vi "HostMain.vi"() -> ()   [LabVIEW 2024]
uses:
  C:/Users/ROAR/Documents/Rob Motor Assessment stuff/Labview/RobUST_3D_with_Unity_Control_PXI_Low_Level_Only_Streamlined/Vicon_files/ViconDataStreamSDK_DotNET.dll
  Vicon_files/ViconDataStreamSDK_DotNET.dll
  typeDef/Modes_knees.ctl
  <vilib>/Platform/TimedLoop/XDataNode/timing_clust.ctl
  <vilib>/Platform/TimedLoop/XDataNode/nitl_modes.ctl
  <vilib>/Platform/TimedLoop/XDataNode/wakeup.ctl
  <vilib>/Utility/file.llb/Read Delimited Spreadsheet (DBL).vi
  <vilib>/platform/TimedLoop/XDataNode/XDataNode.xnode
  <vilib>/Utility/Variable/NI_VariableUtilities.lvlib
  <vilib>/Platform/TimedLoop/XDataNode/XDNodeRunTimeDep.lvlib
  <vilib>/Analysis/NI_AALBase.lvlib
panel:
  out "All tensions mean":dbl[](array[numeric])
  out "Captured tensions mean":dbl[](array[numeric])
  out "Captured tensions standard dev":dbl[](array[numeric])
  in  "Capture current tension mean and standard dev":bool
  out "All tensions standard dev":dbl[](array[numeric])
  out "All tensions history":dbl[][](array[numeric])
  in  "ConstantModeActiveMotorFlags":bool[](array[boolean])
  out "StartManualTensionRecordTimeInSeconds":dbl
  out "RecordTime (s)":dbl
  out "Manually record tensions flag previous state":bool
  in  "MaxTensionsRecordTimeInSecs":dbl
  in  "RecordTensionsForGivenTimeFlag":bool
  out "Task has ended flag":bool
  out "Tension tare values":dbl[](array[numeric])
  in  "Live plot tensions flag":bool
  out "New info string received":bool
  out "Unity task info string":string
  in  "Use sinusoid":bool
  in  "Sinusoid period (s)":dbl
  in  "Sinusoid amplitude (N)":dbl
  in  "Single motor number":i32
  in  "Single motor tension current set value":dbl=10.0 min=10.0
  in  "Single motor tension desired set value":dbl
  in  "Change constant tension value toggle":bool
  out "Finished Late? [i-1]":bool
  out "CablesTared?":bool
  out "Data to save":dbl[][](array[numeric])
  out "Current save file out":path
  out "Connected to Unity last save call?":bool
  in  "Constant mode cable tensions N":dbl
  out "Last Vicon Frame Read":u32
  out "LastTimeUnityTensionsReceivedInMs":u32
  out "TensionsUpdateRateHz":dbl
  out "UnityDesiredCableTensionsInAscendingOrder":dbl[](array[numeric])
  in  "Mode Robot":T1(radio)
  in  "Total Number Motors":i32
  out "Latest tensions":dbl[](array[numeric])
  in  "Tare":bool
  out "Trunk Structure Matrix":dbl[][](array[numeric])
  out "Trunk FF type specifier":string
  out "Center point for FF":dbl[](array[numeric])
  out "Excursion distances Vicon frame":dbl[](array[numeric])
  out "TCP connection to Unity?":bool
  out "Unity TCP connection ID":refnum<k5>
  out "Control point position coords":dbl[](array[numeric])
  in  "Control point data source":T2(radio)
  in  "perturbation directions":string
  in  "Refresh Center 2":bool
  in  "Insert Test Name":string
  out "CurrentPttrunk":cluster{dbl[], dbl[]}
  out "Centertrunk":cluster{dbl[], dbl[]}
  out "xyboundstrunk":cluster{dbl[], dbl[]}
  out "trunk markers":dbl[](array[numeric])
  out "pel markers":dbl[](array[numeric])
  out "whichMode 3":bool[](array[boolean])
  in  "Mode Knees":T3
  out "whichMode 2":bool[](array[boolean])
  in  "?":enum32{"Trunk FF", "Pelvis FF"}(tab)
  in  "Turn On":bool
  out "Trunk Graph":cluster{dbl[], dbl[]}[](graph)
  out "Pelvis Graph":cluster{dbl[], dbl[]}[](graph)
  in  "Turn On Pelv":bool
  out "PelvisGraphyz":cluster{dbl[], dbl[]}[](graph)
  in  "?":T4(tab)
  in  "% Body Weight":dbl=10.0
  in  "FM --- FF":dbl[](array[numeric])=[30.0, 15.0, 15.0, 15.0, 2.0, 2.0]
  in  "Force Field Radius (m)":dbl=0.05
  in  "Update R or FF":bool
  in  "Refresh Center":bool
  in  "Select File with Trunk\nBoundary Points":path=path "" caption="start path"
  in  "Pert Reset":bool
  in  "Apply Pert":bool
  out "Weight [lbs]":dbl
  in  "Update Pert Parameters":bool
  in  "Pert Direction":i16(knob) scale=0.0..7.0
  in  "Rise Time":dbl
  in  "Constant Time":dbl
  in  "Fall Time":dbl
  in  "Amp [%BW]":dbl
  in  "Weight [Kg]":dbl
  in  "Mode Pelvis":enum32{"Idle", "Constant", "Force", "Pert"}(radio)
  out "Boolean":bool
  out "14":cluster{"[0]":dbl, "[1]":dbl}(graph)
  out "13":cluster{"[0]":dbl, "[1]":dbl}(graph)
  out "12":cluster{"[0]":dbl, "[1]":dbl}(graph)
  out "11":cluster{"[0]":dbl, "[1]":dbl}(graph)
  out "10":cluster{"[0]":dbl, "[1]":dbl}(graph)
  out "9":cluster{"[0]":dbl, "[1]":dbl}(graph)
  in  "?":T5(tab)
  in  "Reset Label":bool
  out "Going Up":bool
  in  "record trajectory":bool
  in  "Weight (Kg) --- FF 2":dbl=50.0
  in  "% Body Weight 2":dbl=10.0
  in  "FM --- FF 2":dbl[](array[numeric])=[30.0, 5.0, 5.0, 5.0, 2.0, 2.0]
  in  "Update R or FF 2":bool
  in  "Pelvis Radius FF":dbl=0.03
  in  "Weight [Kg] 3":dbl=75.0
  in  "Amp [%BW] 3":dbl=10.0
  in  "Fall Time 2":dbl=200.0
  in  "Constant Time 2":dbl=200.0
  in  "Rise Time 2":dbl=200.0
  in  "Pert Direction 2":i16(knob) scale=0.0..7.0
  in  "Update Pert Parameters 2":bool
  out "Weight [lbs] 3":dbl
  in  "Apply Pert 2":bool
  in  "Pert Reset 2":bool
  in  "Set Unit Force Vector":dbl[](array[numeric])=[0.0, 0.0, -1.0, 15.0, 2.0, 2.0]
  in  "Update_setForces":bool
  in  "Set % Body Weight":dbl=10.0
  in  "Weight (lb)":dbl=50.0
  out "ATI":dbl[](graph)
  in  "ATI UnBias":bool
  in  "ATI Bias":bool
  out "Saving Data":bool
  out "whichMode":bool[](array[boolean])
  in  "pidGains":dbl[][](array[numeric])=[[3.5, 1.7, 3.0000000000000004, 1.7, 1.7, 3.5, 1.7, 1.7, 2.0, 1.7, 1.7, 3.0, 1.7, 3.5], [0.001, 0.003, 0.003, 0.001, 0.001, 0.003, 0.0008, 0.003, 0.001, 0.003, 0.001, 0.003, 0.001, 0.001], [0.0004, 0.0012, 0.0006, 0.0012, 0.0012, 0.0004, 0.0012, 0.0012, 0.0008, 0.0012, 0.0012, 0.0004, 0.0012, 0.0004]]
  in  "SetPID":bool
  out "4":cluster{"[0]":dbl, "[1]":dbl}(graph)
  out "3":cluster{"[0]":dbl, "[1]":dbl}(graph)
  out "2":cluster{"[0]":dbl, "[1]":dbl}(graph)
  out "1":cluster{"[0]":dbl, "[1]":dbl}(graph)
  out "8":cluster{"[0]":dbl, "[1]":dbl}(graph)
  out "7":cluster{"[0]":dbl, "[1]":dbl}(graph)
  out "6":cluster{"[0]":dbl, "[1]":dbl}(graph)
  out "FB n FF O/P(N)":dbl[](graph)
  out "Current Filename":string
  out ".NET Reference out":refnum<k24>
  out "ViconTab":enum32{"Vicon", "no Vicon"}(tab)
  out "Frame Number":dbl format="%.2f"
  out "Subject Name":string
  out "Markers Count":u32
  in  "Connect\nVicon":bool
  in  "Update\nMarkers":bool
  in  "Vicon Static":bool
  in  "Stream Mode":i32(ring) items=["ClientPull", "ClientPullPreFetch", "ServerPush"]
  out "SDK Version":string
  out "Vicon Connected":bool
  out "5":cluster{"[0]":dbl, "[1]":dbl}(graph)
  out "Voltage O/P (V)":dbl[](graph)
  in  "Use ATI":bool
  in  "ATIDAQFT._FTSensor":refnum<k7>
  in  "UseVicon":bool
  out "Loop Durations (uSec)":i64[](array[numeric])
  in  "DataSave":bool
  in  "Stop":bool
  # "Notes on running HostMain.vi\n1.)  Start  HostMain (auto in Unity control point mode, Idle Trunk mode).\n2.) Then start targetController.vi (for now)\n3.) The tension sensors MUST be tared when the trunk is in  Idle mode.\n4.) Live tension sensor plots are directly below this text! (scroll down)"
  # "STAND TRAINER\n                     Software developed by Vineet Vashista (2014), Moiz Khan (2016-19), Tatiana Luna (2019-20)"
  # "Unity Communication Info Panel"
  # "TCP Connection Status"
  # "General Robot Constants\n(Set in code)"
  # "Current Unity task information string"
  # "Pelvis-Planar"
  # "Data received from Unity (old, deprecated, could delete!)"
  # "Key coordinates"
  # "----->"
  # "Tare tension sensors panel\nNOTE: tare only works in \nRobotMode = Idle"
  # "Manually start tension recording\n(Note: auto-start with Unity messages\nis typical)"
  # "Robot control panel"
  # "2                          3                                           4                                  5                                      6                        7                                  8                           9                                    10                               11                            12                              13                                   14"
  # "HAVE TO TARE\nBEFORE ROBOT\nMODES BECOME\nENABLED!"
  # "Excursion distance measurements"
  # "Constant mode control"
  # "Single motor mode step change"
  # "Motor 1"
  # "Motor 2"
  # "Motor 3"
  # "Motor 4"
  # "Motor 5"
  # "Motor 6"
  # "Motor 7"
  # "Motor 8"
  # "Motor 9"
  # "FF mode type specifier"
  # "Motor 10"
  # "Types: \"I\" = idle; \"B\" = excursion \nboundary 2D"
  # "Motor 11"
  # "Motor 12"
  # "Motor 13"
  # "Motor 14"
  # "PELVIS TOP MOTORS"
  # "TRUNK MOTOR CABLE \nTENSIONS [N]"
  # "Sensor ID: FT5769"
  # "Mx(Nm)"
  # "My(Nm)"
  # "Mz(Nm)"
  # "PID                   QP                  File"
  # "This can be changed only starting of host"
  # "Pelvis-Moments"
  # "PELVIS BOTTOM MOTORS"
  # "SHANK MOTOR CABLE TENSIONS [N]"
  # "Circular Force Field"
  # "Irregular Force Field"
  # "Fz\nMx\nMy\nMz"
  # "30,15,15,15"
  # "Pert Parameters"
  # "FIRST PERT GIVEN BY\nCLICKING TURN ON PERT!!!"
  # "Pert Parameters"
  # "FIRST PERT GIVEN BY\nCLICKING TURN ON PERT!!!"
  # "X\n\nY\n\nZ"
  # "Trunk Static"
  # "Pelvis Static"
  # "Set Tension = Mag + Constant Tension + Step"
  # "TRUNK CONTROL"
  # "PELVIS CONTROL"
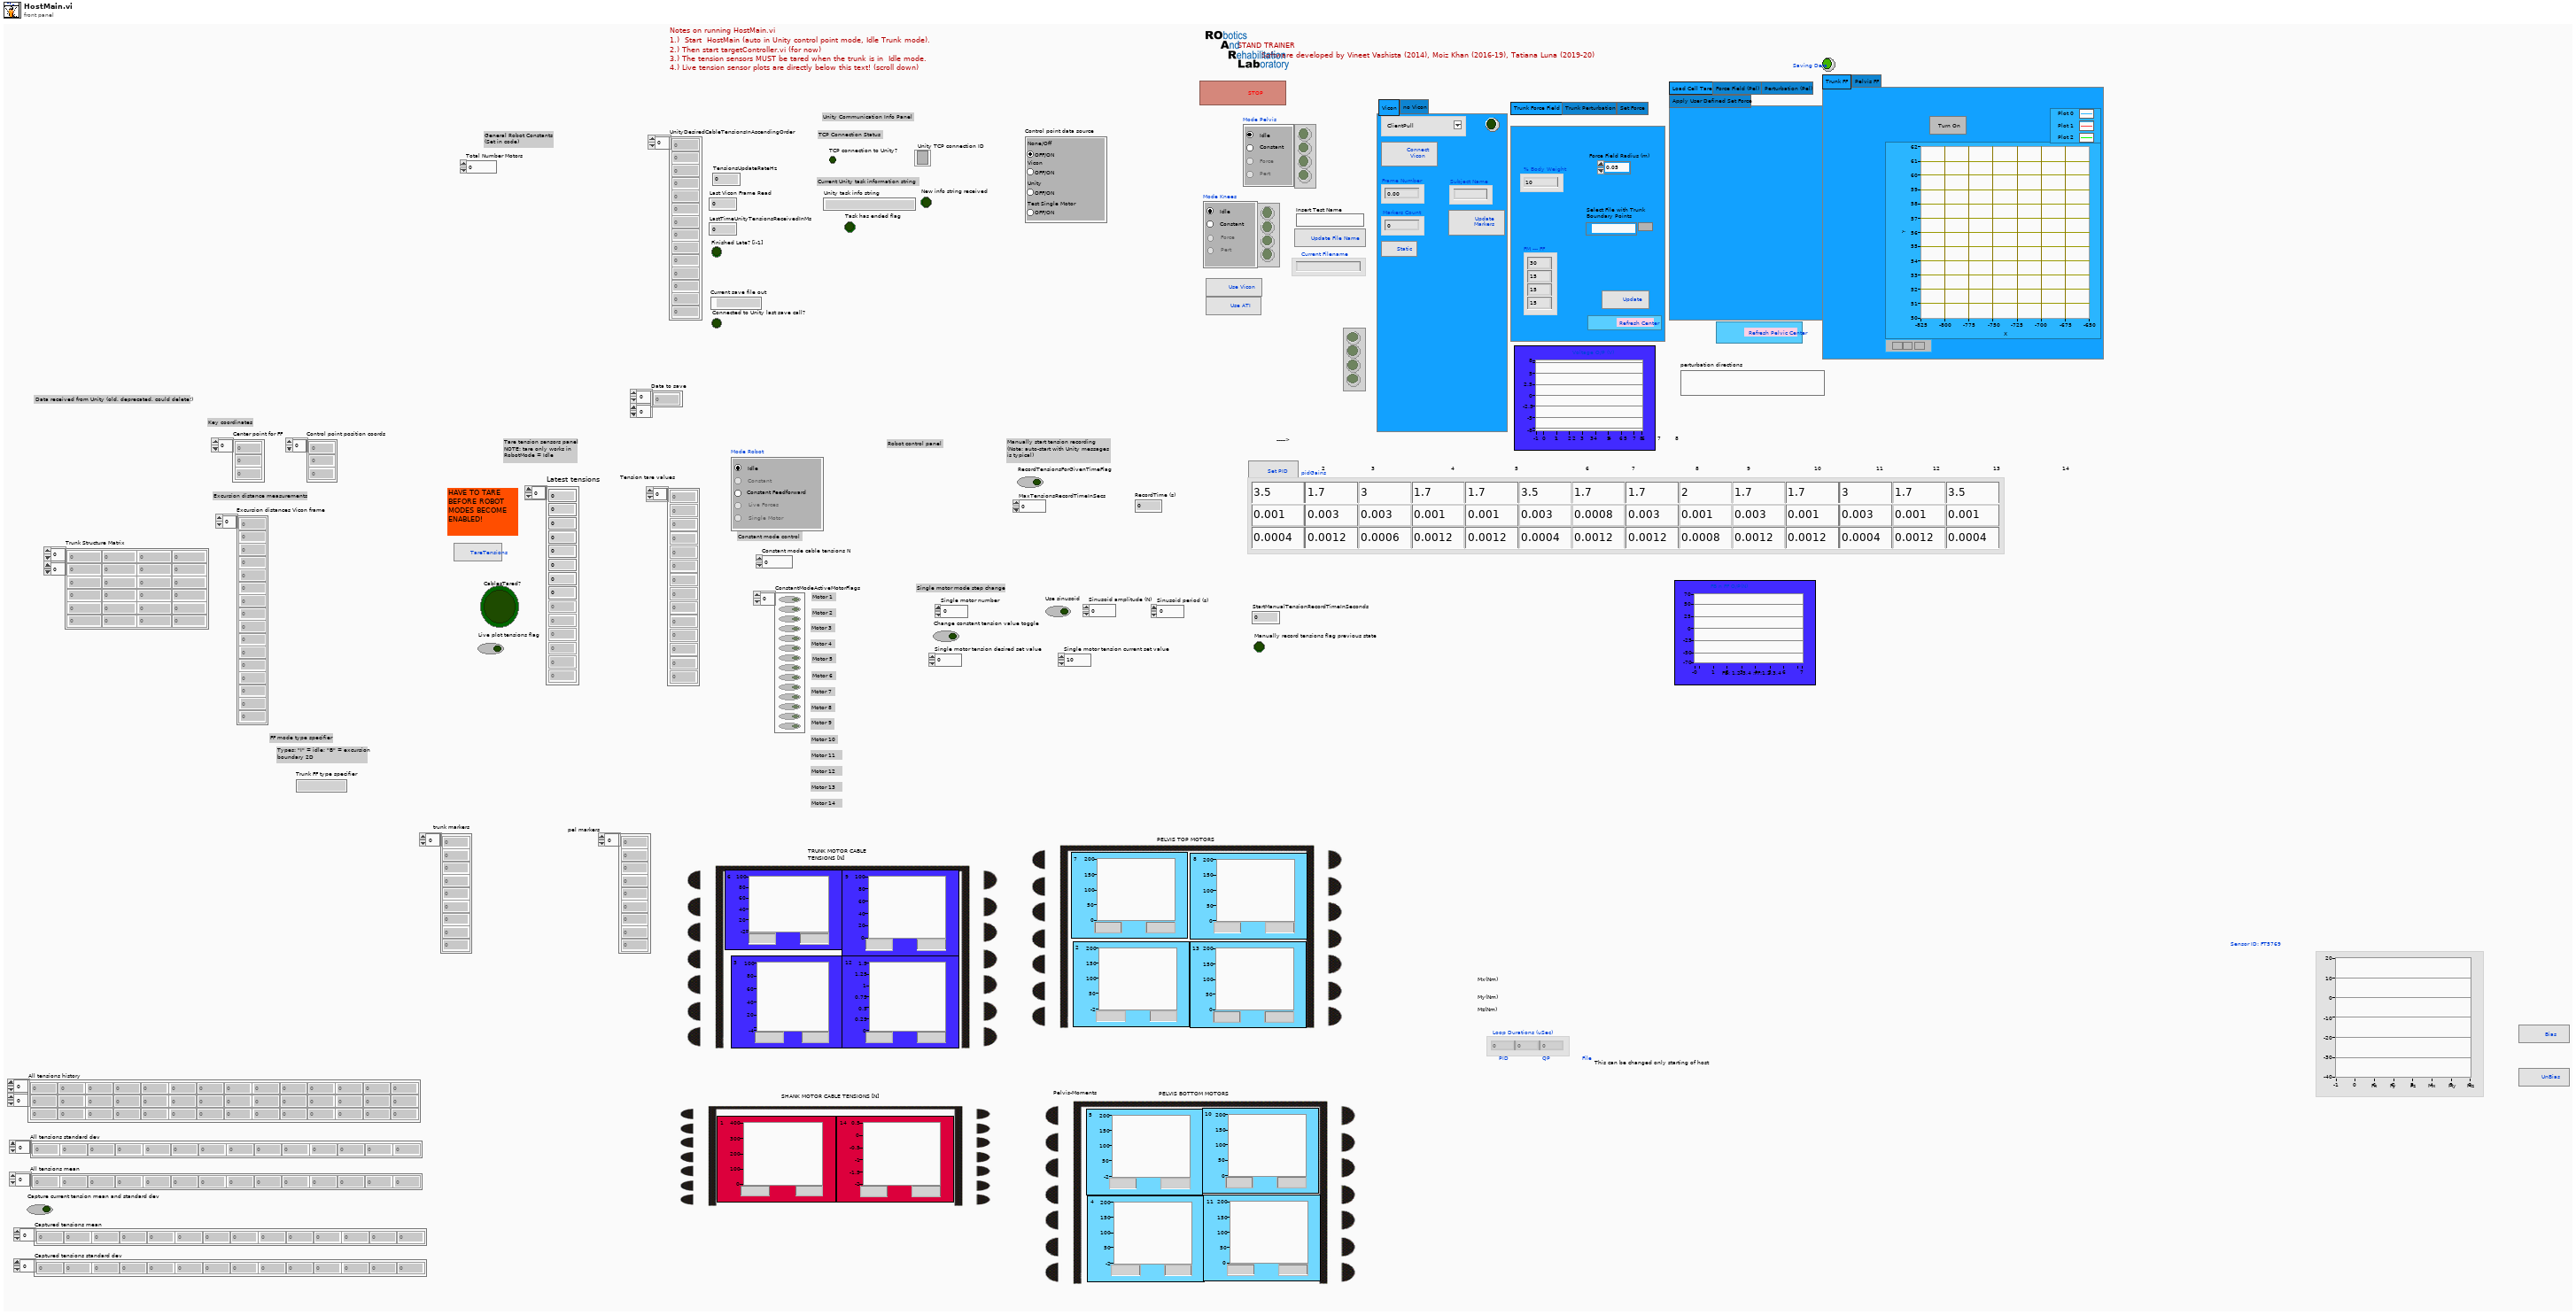
[diagram p1: front panel]
types:
  T1 = enum32{"Idle", "Constant", "Live Forces", "Single Motor", "Constant Feedforward"}
  T2 = enum32{"None/Off", "Vicon", "Unity", "Test Single Motor"}
  T3 = typedef "Modes_knees.ctl" = enum32{"Idle", "Constant", "Force", "Pert"}
  T4 = enum32{"Trunk Force Field", "Trunk Perturbation", "Set Force"}
  T5 = enum32{"Load Cell Tare", "Force Field (Pel)", "Perturbation (Pel)", "Apply User Defined Set Force"}
  T6 = enum32{"Idle", "Constant", "Live Forces", "Single Motor"}
  T7 = enum8{"Enabled", "Disabled", "Disabled and Grayed Out"}
  T8 = typedef "XDNodeRunTimeDep.lvlib/timing_clust.ctl" = cluster{"Expected End [f-1]":u64, "Actual End [f-1]":u64, "Finished Late? [f-1]":bool, "Expected End [i-1]":u64, "Actual End [i-1]":u64, "Finished Late? [i-1]":bool, "Expected Start [i]":u64, "Actual Start [i]":u64, "Expected Start [f]":u64, "Actual Start [f]":u64, "Source Name":string, "Structure Name":string, "Period":i64, "Deadline":i64, "Offset":i64, "Start":i64, "Priority":i32, "Timeout":i32, "Mode":T9, "Wakeup Reason":T10, "Error":errorcluster, "Source Type":string, "Secondary Source Type":string, "Global End Time":u64, "Global Start Time":u64, "Frame Duration":u64, "Iteration Duration":u64, "Assigned CPU":i32, "I/O Scan Engine Mode":u32}
  T9 = typedef "XDNodeRunTimeDep.lvlib/nitl_modes.ctl" = enum32{"No Change", "Process missed periods, maintain original phase", "Discard missed periods, maintain original phase", "Process missed periods, ignore original phase", "Discard missed periods, ignore original phase"}
  T10 = typedef "XDNodeRunTimeDep.lvlib/wakeup.ctl" = enum32{"Normal", "Aborted", "Asynchronous wakeup", "Timing source error", "Timed loop error", "Timeout"}
  T11 = enum16{"Standard", "Buffered", "CRLF", "Immediate"}
  T12 = cluster{"Most Recent Vicon Frame Number":u32, "Corresponding motor tensions":dbl[], "Motor numbers":i32[]}
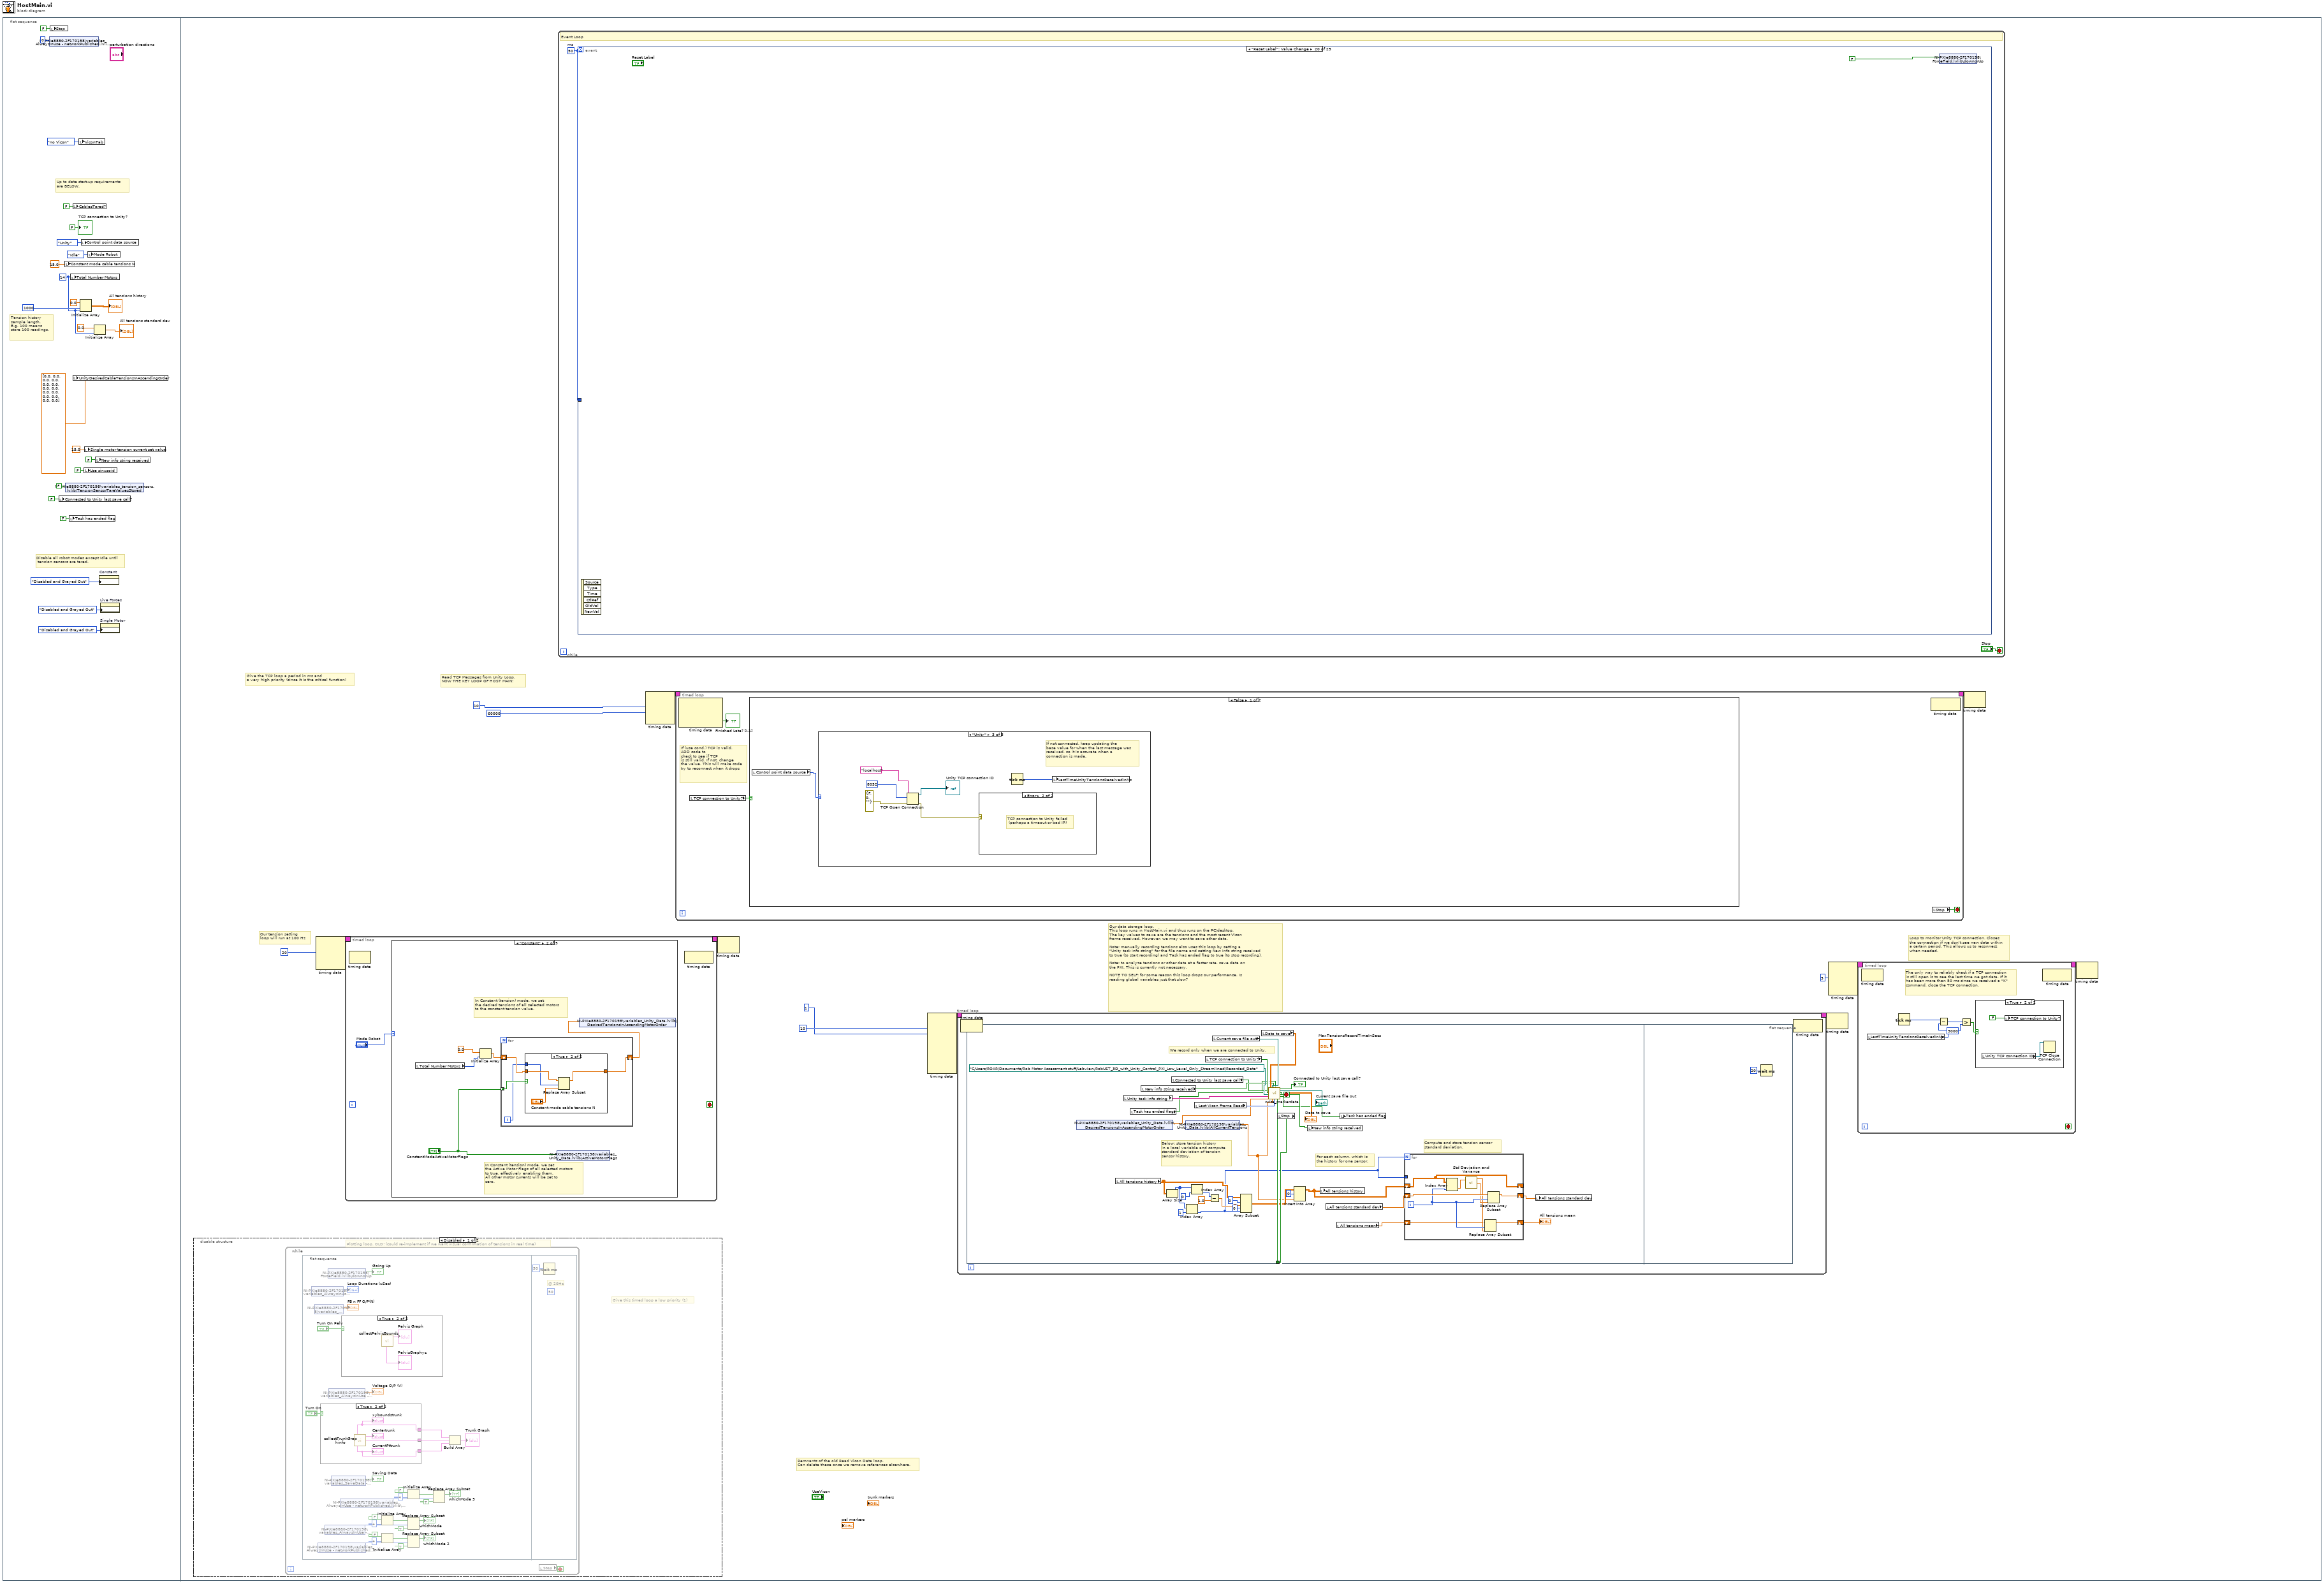
[diagram p0: block diagram]
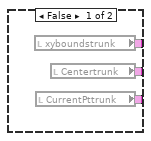
[diagram p3: hidden frame]
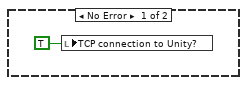
[diagram p8: hidden frame]
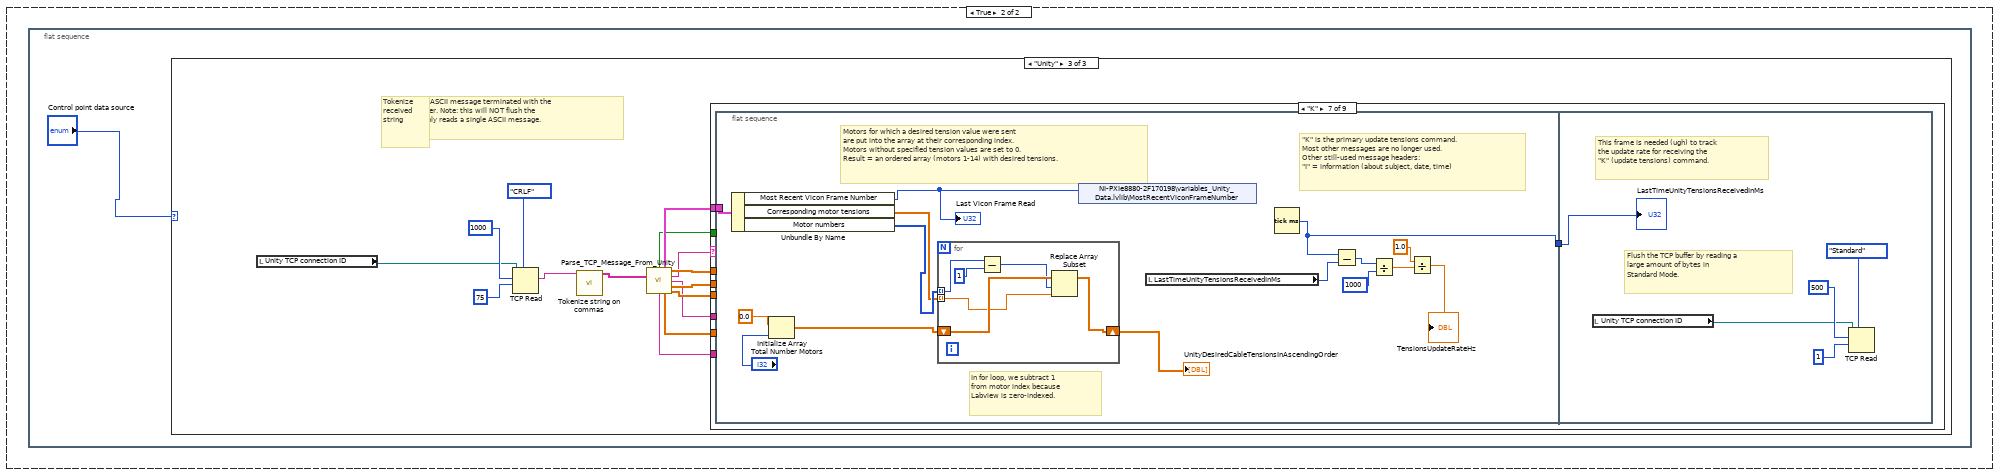
[diagram p9: hidden frame]
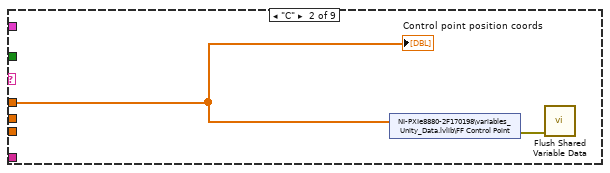
[diagram p13: hidden frame]
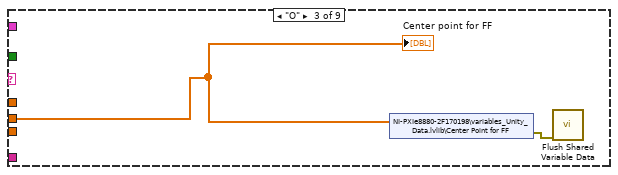
[diagram p14: hidden frame]
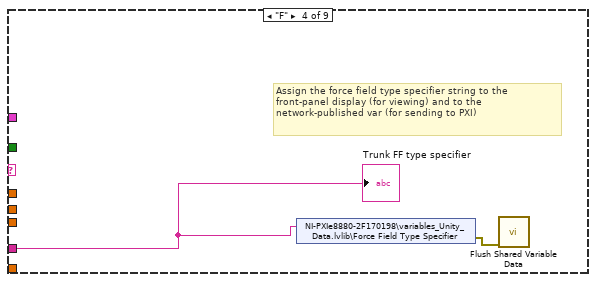
[diagram p15: hidden frame]
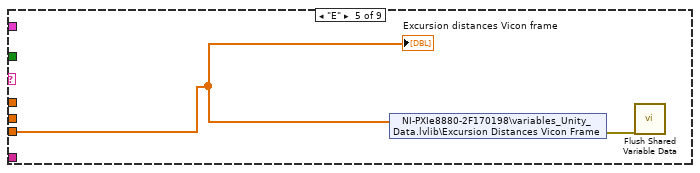
[diagram p16: hidden frame]
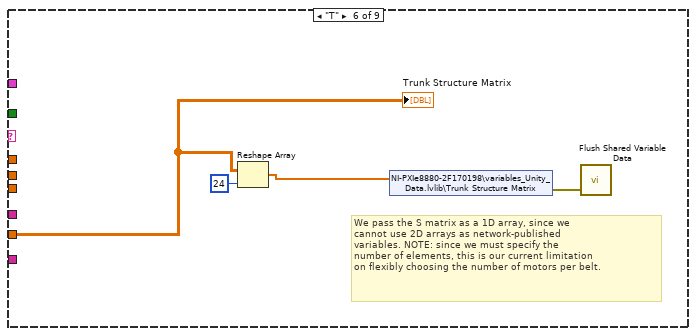
[diagram p17: hidden frame]
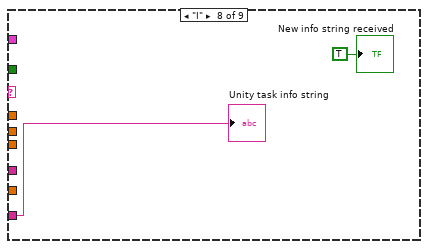
[diagram p18: hidden frame]
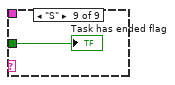
[diagram p19: hidden frame]
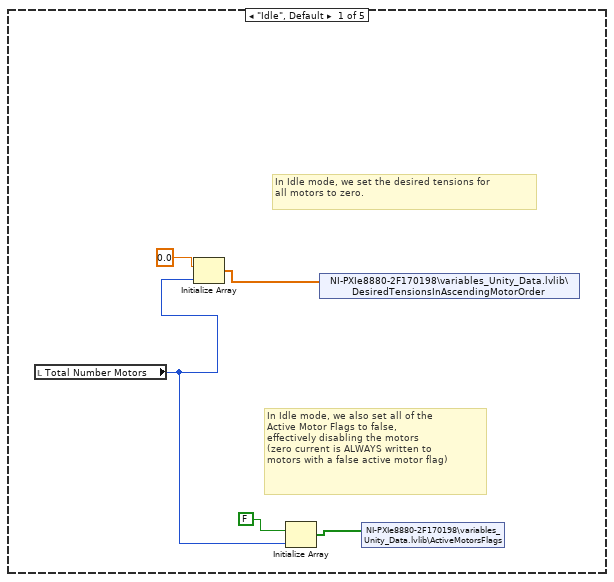
[diagram p20: hidden frame]
diagram:
  n1 = flat-sequence {
    frame #0 {
      w3 = 14 ("Total Number Motors")
      # "Tension history \nsample length. \nE.g. 100 means \nstore 100 readings."
      # "Disable all robot modes except Idle until\n tension sensors are tared."
      # "Up to date start-up requirements\nare BELOW."
      n2 = shared-variable "NI-PXIe8880-2F170198\\variables_AlwaysInUse - networkPublished.lvlib\\Trunk Belt Mode"(i16 0 ("Mode")) -> ()  [unwired: 1 in, 1 out]
      n3 = local write "Stop"(FALSE ("Force")) -> ()
      n4 = local write "Connected to Unity last save call?"(FALSE ("Connected to Unity last save call?")) -> ()
      n5 = local write "Constant mode cable tensions N"(15.0 ("Constant mode cable tensions (N)")) -> ()
      n6 = shared-variable "NI-PXIe8880-2F170198\\variables_tension_sensors.lvlib\\TensionSensorTareValuesStored"(FALSE ("TensionSensorTareValuesStored")) -> ()  [unwired: 1 in, 1 out]
      n7 = local write "Task has ended flag"(FALSE ("Task has ended flag")) -> ()
      n8 = local write "Total Number Motors"(w3) -> ()
      n9 = local write "CablesTared?"(FALSE ("CablesTared?")) -> ()
      n10 = local write "UnityDesiredCableTensionsInAscendingOrder"(dbl[] [0.0, 0.0, 0.0, 0.0, 0.0, 0.0, 0.0, 0.0, 0.0, 0.0, 0.0, 0.0, 0.0, 0.0] ("UnityDesiredCableTensionsInAscendingOrder")) -> ()
      n11 = local write "ViconTab"(enum32{"Vicon", "no Vicon"}."no Vicon" ("ViconTab")) -> ()
      n12 = Initialize Array(0.0 ("element"), 1000 ("dimension size"), w3) -> (→"All tensions history":dbl[][])
      n13 = local write "Control point data source"(enum32{"None/Off", "Vicon", "Unity"}."Unity" ("Control point data source")) -> ()
      n14 = local write "Use sinusoid"(FALSE ("Use sinusoid")) -> ()
      n15 = local write "Single motor tension current set value"(15.0 ("Single motor tension current set value")) -> ()
      n16 = local write "Mode Robot"(T6."Idle" ("Mode Robot")) -> ()
      n17 = Initialize Array(0.0 ("element"), w3) -> (→"All tensions standard dev":dbl[])
      n18 = local write "New info string received"(FALSE ("New info string received")) -> ()
      n19 = property on="Constant" class="Bool (strict)"("DisabledEnum"=T7."Disabled and Grayed Out" ("Disabled")) -> ()  [unwired: 2 in, 2 out]
      n20 = property on="Live Forces" class="Bool (strict)"("DisabledEnum"=T7."Disabled and Grayed Out" ("Disabled")) -> ()  [unwired: 2 in, 2 out]
      n21 = property on="Single Motor" class="Bool (strict)"("DisabledEnum"=T7."Disabled and Grayed Out" ("Disabled")) -> ()  [unwired: 2 in, 2 out]
      "TCP connection to Unity?" <- FALSE ("TCP connection to Unity?")
    }
    frame #1 {
      # "Our data storage loop. \nThis loop runs in HostMain.vi and thus runs on the PC/desktop. \nThe key values to save are the tensions and the most recent Vicon \nframe received. However, we may want to save other data.\n\nNote: manually recording tensions also uses this loop by setting a \n\"Unity task info string\" for the file name and setting New info string received\nto true (to start recording) and Task has ended flag to true (to stop recording). \n\nNote: to analyze tensions or other data at a faster rate, save data on \nthe PXI. This is currently not necessary.\n\nNOTE TO SELF: for some reason this loop drops our performance. Is\nreading global variables just that slow?"
      # "Loop to monitor Unity TCP connection. Closes\nthe connection if we don't see new data within\na certain period. This allows us to reconnect \nwhen needed."
      # "Remnants of the old Read Vicon Data loop. \nCan delete these once we remove references elsewhere."
      # "Give the TCP loop a period in ms and \na very high priority (since it is the critical function)"
      # "Our tension setting\nloop will run at 100 Hz"
      # "Read TCP Messages from Unity Loop. \nNOW THE KEY LOOP OF HOST MAIN!"
      n22 = disable-structure shown="Disabled" {
        frame Disabled {
          # "Give this timed loop a low priority (1)"
          # "Plotting loop. OLD! (could re-implement if we want visual confirmation of tensions in real time)"
          n23 = while {
            stop <- w91 stop-if-true
            n24 = flat-sequence {
              frame #0 {
                n25 = shared-variable "NI-PXIe8880-2F170198\\variables_AlwaysInUse - networkPublished.lvlib\\timings"() -> (→"Loop Durations (uSec)":i64[])  [unwired: 1 in, 1 out]
                n26 = shared-variable "NI-PXIe8880-2F170198\\variables_AlwaysInUse - networkPublished.lvlib\\FBnFF"() -> (→"FB n FF O/P(N)":dbl[])  [unwired: 1 in, 1 out]
                n27 = shared-variable "NI-PXIe8880-2F170198\\variables_AlwaysInUse - networkPublished.lvlib\\whichMode_pel"() -> (w105:i16)  [unwired: 1 in, 1 out]
                n28 = case shown="True" "Turn On" {
                  tunnel: [w125 w128] -> w97
                  tunnel: [w124 w127] -> w96
                  tunnel: [w123 w126] -> w95
                  frame False {
                    n29 = local read "xyboundstrunk"() -> (w125:cluster{dbl[], dbl[]})
                    n30 = local read "CurrentPttrunk"() -> (w123:cluster{dbl[], dbl[]})
                    n31 = local read "Centertrunk"() -> (w124:cluster{dbl[], dbl[]})
                  }
                  frame True {
                    n32 = call "collectTrunkGraphinfo.vi"() -> ("CurrentPttrunk"=w126:cluster{dbl[], dbl[]}, "Centertrunk"=w127:cluster{dbl[], dbl[]}, "xyboundstrunk"=w128:cluster{dbl[], dbl[]})  [unwired: 3 in]
                    "xyboundstrunk" <- w128
                    "Centertrunk" <- w127
                    "CurrentPttrunk" <- w126
                  }
                }
                n33 = shared-variable "NI-PXIe8880-2F170198\\variables_AlwaysInUse - networkPublished.lvlib\\whichMode"() -> (w118:i16)  [unwired: 1 in, 1 out]
                n34 = shared-variable "NI-PXIe8880-2F170198\\ForceField.lvlib\\downorUp"() -> (→"Going Up":bool)  [unwired: 1 in, 1 out]
                n35 = shared-variable "NI-PXIe8880-2F170198\\variables_AlwaysInUse - networkPublished.lvlib\\op2Motor"() -> (→"Voltage O/P (V)":dbl[])  [unwired: 1 in, 1 out]
                n36 = shared-variable "NI-PXIe8880-2F170198\\variables_SaveData - networkPublished.lvlib\\SaveData"() -> (→"Saving Data":bool)  [unwired: 1 in, 1 out]
                n37 = shared-variable "NI-PXIe8880-2F170198\\variables_AlwaysInUse - networkPublished.lvlib\\whichMode_knees"() -> (w103:i16)  [unwired: 1 in, 1 out]
                n38 = case shown="True" "Turn On Pelv" {
                  frame False {
                  }
                  frame True {
                    n39 = call "collectPelvicBounds.vi"() -> ("yzgraph array"=→"PelvisGraphyz":cluster{dbl[], dbl[]}[], "xzgraph"=→"Pelvis Graph":cluster{dbl[], dbl[]}[])  [unwired: 10 in]
                  }
                }
                n40 = Initialize Array(FALSE ("Force"), 4 ("dimension size")) -> (w117:bool[])
                n41 = Initialize Array(FALSE ("Force"), 4 ("dimension size")) -> (w109:bool[])
                n42 = Initialize Array(FALSE ("Force"), 4 ("dimension size")) -> (w102:bool[])
                n43 = Replace Array Subset(array=w117, new element=TRUE ("Force"), index=w118) -> (→"whichMode":bool[])
                n44 = Replace Array Subset(array=w109, new element=TRUE ("Force"), index=w105) -> (→"whichMode 2":bool[])
                n45 = Replace Array Subset(array=w102, new element=TRUE ("Force"), index=w103) -> (→"whichMode 3":bool[])
                n46 = Build Array(w97, w96, w95) -> (→"Trunk Graph":cluster{dbl[], dbl[]}[])
              }
              frame #1 {
                (unwired) u32 50 ("milliseconds to wait")
                # "@ 20Hz"
                n47 = Wait (ms)(milliseconds to wait=u32 50) -> ()  [unwired: 1 out]
              }
            }
            n48 = local read "Stop"() -> (w91:bool)
          }
        }
        frame Enabled {
        }
      }
      n49 = node-c288(i64 20 ("Period")) -> (w38:T8)  [unwired: 3 in]
      n50 = timed-loop {
        timing: w38 -> [_]
        timing-out: [_] -> w37
        stop <- _ stop-if-true
        n51 = node-c288() -> ()  [unwired: 1 in, 1 out]
        n52 = case shown="\"Constant\"" "Mode Robot" {
          frame "Idle", Default {
            # "In Idle mode, we also set all of the \nActive Motor Flags to false, \neffectively disabling the motors \n(zero current is ALWAYS written to \nmotors with a false active motor flag)"
            # "In Idle mode, we set the desired tensions for\nall motors to zero."
            n53 = local read "Total Number Motors"() -> (w223:i32)
            n54 = Initialize Array(0.0 ("element"), w223) -> (w225:dbl[])
            n55 = Initialize Array(FALSE, w223) -> (w222:bool[])
            n56 = shared-variable "NI-PXIe8880-2F170198\\variables_Unity_Data.lvlib\\DesiredTensionsInAscendingMotorOrder"(w225) -> ()  [unwired: 1 in, 1 out]
            n57 = shared-variable "NI-PXIe8880-2F170198\\variables_Unity_Data.lvlib\\ActiveMotorsFlags"(w222) -> ()  [unwired: 1 in, 1 out]
          }
          frame "Constant" {
            # "In Constant (tension) mode, we set\nthe Active Motor Flags of all selected motors\nto true, effectively enabling them. \nAll other motor currents will be set to \nzero."
            # "In Constant (tension) mode, we set\nthe desired tensions of all selected motors\nto the constant tension value."
            n58 = local read "Total Number Motors"() -> (w231:i32)
            n59 = Initialize Array(0.0 ("element"), w231) -> (w229:dbl[])
            n60 = for {
              tunnel: "ConstantModeActiveMotorFlags" -> [w235] mode=indexing
              shift-right: [w233] -> w228
              shift-left: w229 -> [w234]
              i -> [w232]
              n61 = case shown="True" w235 {
                tunnel: w234 -> [w236 w239]
                tunnel: [w236 w238] -> w233
                tunnel: w232 -> [_ w237]
                frame False {
                }
                frame True {
                  n62 = Replace Array Subset(array=w239, new element="Constant mode cable tensions N", index=w237) -> (w238:dbl[])
                }
              }
            }
            n63 = shared-variable "NI-PXIe8880-2F170198\\variables_Unity_Data.lvlib\\ActiveMotorsFlags"("ConstantModeActiveMotorFlags") -> ()  [unwired: 1 in, 1 out]
            n64 = shared-variable "NI-PXIe8880-2F170198\\variables_Unity_Data.lvlib\\DesiredTensionsInAscendingMotorOrder"(w228) -> ()  [unwired: 1 in, 1 out]
          }
          frame "Constant Feedforward" {
            # "In Constant (tension) mode, we set\nthe Active Motor Flags of all selected motors\nto true, effectively enabling them. \nAll other motor currents will be set to \nzero."
            # "In Constant (tension) mode, we set\nthe desired tensions of all selected motors\nto the constant tension value."
            n65 = local read "ConstantModeActiveMotorFlags"() -> (w241:bool[])
            n66 = local read "Total Number Motors"() -> (w245:i32)
            n67 = Initialize Array(0.0 ("element"), w245) -> (w243:dbl[])
            n68 = for {
              tunnel: w241 -> [w249] mode=indexing
              shift-right: [w247] -> w242
              shift-left: w243 -> [w248]
              i -> [w246]
              n69 = case shown="True" w249 {
                tunnel: w248 -> [w250 w254]
                tunnel: [w250 w253] -> w247
                tunnel: w246 -> [_ w252]
                frame False {
                }
                frame True {
                  n70 = local read "Constant mode cable tensions N"() -> (w251:dbl)
                  n71 = Replace Array Subset(array=w254, new element=w251, index=w252) -> (w253:dbl[])
                }
              }
            }
            n72 = shared-variable "NI-PXIe8880-2F170198\\variables_Unity_Data.lvlib\\ActiveMotorsFlags"(w241) -> ()  [unwired: 1 in, 1 out]
            n73 = shared-variable "NI-PXIe8880-2F170198\\variables_Unity_Data.lvlib\\DesiredTensionsInAscendingMotorOrder"(w242) -> ()  [unwired: 1 in, 1 out]
          }
          frame "Live Forces" {
            # "In Live Forces mode, we set\nthe active flag of all motors\n that have non-zero desired \ntensions to true, effectively\nenabling them."
            n74 = local read "UnityDesiredCableTensionsInAscendingOrder"() -> (w259:dbl[])
            n75 = local read "Total Number Motors"() -> (w258:i32)
            n76 = Initialize Array(FALSE, w258) -> (w256:bool[])
            n77 = for {
              tunnel: w259 -> [w266] mode=indexing
              shift-right: [w261] -> w255
              shift-left: w256 -> [w262]
              i -> [w260]
              n78 = Equal?(x=w266, y=0.0) -> (x = y?=w264:bool)
              n79 = Not(x=w264) -> (.not. x?=w263:bool)
              n80 = case shown="True" w263 {
                tunnel: w262 -> [w267 w271]
                tunnel: [w267 w268] -> w261
                tunnel: w260 -> [_ w269]
                frame False {
                }
                frame True {
                  n81 = Replace Array Subset(array=w271, new element=TRUE ("new element/subarray"), index=w269) -> (w268:bool[])
                }
              }
            }
            n82 = shared-variable "NI-PXIe8880-2F170198\\variables_Unity_Data.lvlib\\DesiredTensionsInAscendingMotorOrder"(w259) -> ()  [unwired: 1 in, 1 out]
            n83 = shared-variable "NI-PXIe8880-2F170198\\variables_Unity_Data.lvlib\\ActiveMotorsFlags"(w255) -> ()  [unwired: 1 in, 1 out]
          }
          frame "Single Motor" {
            # "Only one motor is flagged as \nactive in Single Motor control\nmode. All other motor currents\nwill be set to zero."
            # "Subtract 1 b/c of \nzero-indexing"
            n84 = local read "Total Number Motors"() -> (w277:i32)
            n85 = Subtract(x="Single motor number", y=1) -> (x-y=w274:i32)
            n86 = local read "Tension tare values"() -> (w278:dbl[])
            n87 = Initialize Array(FALSE, w277) -> (w275:bool[])
            n88 = Replace Array Subset(array=w275, new element=TRUE ("new element/subarray"), index=w274) -> (w272:bool[])
            n89 = Replace Array Subset(array=w278, new element="Single motor tension current set value", index=w274) -> (w282:dbl[])
            n90 = shared-variable "NI-PXIe8880-2F170198\\variables_Unity_Data.lvlib\\DesiredTensionsInAscendingMotorOrder"(w282) -> ()  [unwired: 1 in, 1 out]
            n91 = shared-variable "NI-PXIe8880-2F170198\\variables_Unity_Data.lvlib\\ActiveMotorsFlags"(w272) -> ()  [unwired: 1 in, 1 out]
          }
        }
        n92 = node-c288() -> ()  [unwired: 1 in, 1 out]
      }
      n93 = while {
        stop <- "Stop" stop-if-true
        w289 = 50  # ms
        # "Event Loop"
        n94 = event shown="[19] \"Reset Label\": Value Change" {
          selector: _ -> [_ _ _ _ _ _ _ _ _ _ _ _ _ _ _ _ _ _ _ _ _ _ _ _ _]
          dyn-events: _ -> [_ _ _ _ _ _ _ _ _ _ _ _ _ _ _ _ _ _ _ _ _ _ _ _ _]
          timeout: w289 -> [_ _ _ _ _ _ _ _ _ _ _ _ _ _ _ _ _ _ _ _ _ _ _ _ _]
          tunnel: w289 -> [w301 _ _ _ _ _ _ _ _ _ _ _ _ _ _ _ _ _ _ _ _ _ _ _ _]
          event Timeout {
            # "If the button for capturing the current tension standard deviation \nis being pressed, store whatever the current values are. \nUsing a \"switch-until-released\" mechanical action on \nthe capture button means a click will just capture the current values."
            # "This block handles manually recording the cable tensions (usually for single motor testing)"
            # "If we want to \nlive-plot the \ntension values"
            # "This event runs every time the timeout period expires. \nSo, since buttons are rarely pressed, it runs quite often.\nUse this event to update states of variables (e.g. mode \nchanges) in a non-urgent way."
            # "On timeout (every 50 ms, if no button presses), \nupdate the robot mode."
            # "THIS CASE STRUCTURE:\n- Reads ATI F/T data, if \nusing"
            # "THIS CASE STRUCTURE:\n- Allows us to (manually?)\nset the PID gains if desired."
            # "THIS CASE STRUCTURE: \n- Tare tension sensors \nin robot mode \"Idle\" only."
            n95 = event-data() -> ()  [unwired: 1 in, 3 out]
            n96 = local read "Single motor number"() -> (w295:i32)
            n97 = local read "Mode Robot"() -> (w296:T1)
            n98 = disable-structure shown="Disabled" {
              frame Disabled {
              }
              frame Enabled {
              }
            }
            n99 = Divide(x=w301, y=1000.0) -> (x/y=w299:dbl)
            n100 = shared-variable "NI-PXIe8880-2F170198\\variables_Unity_Data.lvlib\\RobotControlModeAsInt"(w296) -> ()  [unwired: 1 in, 1 out]
            n101 = shared-variable "NI-PXIe8880-2F170198\\variables_Unity_Data.lvlib\\SingleMotorControlModeMotorNumber"(w295) -> ()  [unwired: 1 in, 1 out]
            n102 = property class="WFChart (strict)"("XScale.Multiplier"=w299) -> ()  [unwired: 2 in, 2 out]
            n103 = case shown="False" "Use ATI" {
              frame False {
              }
              frame True {
                n104 = shared-variable "NI-PXIe8880-2F170198\\variables_ATI - networkPublished.lvlib\\ATI_FM"() -> (→"ATI":dbl[])  [unwired: 1 in, 1 out]
              }
            }
            n105 = case shown="False" "SetPID" {
              selector: "SetPID" -> [_ w400]
              frame False {
              }
              frame True {
                n106 = shared-variable "NI-PXIe8880-2F170198\\variables_ToSetPID - networkPublished.lvlib\\SetPID"(w400) -> ()  [unwired: 1 in, 1 out]
                n107 = Transpose 2D Array(2D array="pidGains") -> (transposed array=w398:dbl[][])
                n108 = Reshape Array(w398, 42 ("dimension size")) -> (w397:dbl[])
                n109 = shared-variable "NI-PXIe8880-2F170198\\variables_ToSetPID - networkPublished.lvlib\\pidGains"(w397) -> ()  [unwired: 1 in, 1 out]
              }
            }
            n110 = shared-variable "NI-PXIe8880-2F170198\\variables_Unity_Data.lvlib\\DesiredTensionsInAscendingMotorOrder"() -> (w297:dbl[])  [unwired: 1 in, 1 out]
            n111 = shared-variable "NI-PXIe8880-2F170198\\variables_Unity_Data.lvlib\\AllCurrentTensions"() -> (w292:dbl[])  [unwired: 1 in, 1 out]
            "Latest tensions" <- w292
            n112 = local read "Mode Robot"() -> (w302:T1)
            n113 = case shown="\"Idle\", Default" w302 {
              frame "Idle", Default {
                # "Load Cell Tare"
                n114 = shared-variable "NI-PXIe8880-2F170198\\variables_tension_sensors.lvlib\\TensionSensorTareValuesStored"() -> (w402:bool)  [unwired: 1 in, 1 out]
                n115 = case shown="True" "Tare" {
                  selector: "Tare" -> [_ w414]
                  tunnel: [w411 w413] -> w404
                  tunnel: [FALSE w414] -> w403
                  frame False {
                    n116 = local read "Tension tare values"() -> (w411:dbl[])
                  }
                  frame True {
                    n117 = local read "Latest tensions"() -> (w413:dbl[])
                    "Tension tare values" <- w413
                    "Boolean" <- w414
                  }
                }
                n118 = case shown="True" w402 {
                  frame False {
                  }
                  frame True {
                    # "If the PXI has tared\nthe tension sensor values,\nenable other robot modes."
                    n119 = property on="Idle" class="Bool (strict)"("DisabledEnum"=T7."Enabled" ("Disabled")) -> ()  [unwired: 2 in, 2 out]
                    n120 = property on="Constant" class="Bool (strict)"("DisabledEnum"=T7."Enabled" ("Disabled")) -> ()  [unwired: 2 in, 2 out]
                    n121 = property on="Live Forces" class="Bool (strict)"("DisabledEnum"=T7."Enabled" ("Disabled")) -> ()  [unwired: 2 in, 2 out]
                    n122 = property on="Single Motor" class="Bool (strict)"("DisabledEnum"=T7."Enabled" ("Disabled")) -> ()  [unwired: 2 in, 2 out]
                    "CablesTared?" <- TRUE ("CablesTared?")
                  }
                }
                n123 = shared-variable "NI-PXIe8880-2F170198\\Load Cell Tare.lvlib\\TareTrue"(w403) -> ()  [unwired: 1 in, 1 out]
                n124 = shared-variable "NI-PXIe8880-2F170198\\Load Cell Tare.lvlib\\Loadcelltare"(w404) -> ()  [unwired: 1 in, 1 out]
              }
              frame "Constant" {
              }
              frame "Live Forces" {
              }
              frame "Single Motor" {
                n125 = case shown="True" "Use sinusoid" {
                  frame False {
                  }
                  frame True {
                    n126 = local read "Single motor tension desired set value"() -> (w418:dbl)
                    n127 = Multiply(x=2.0, y=3.141592653589793) -> (x*y=w424:dbl)
                    n128 = Tick Count (ms)() -> (millisecond timer value=w427:u32)
                    n129 = Divide(x=w427, y=1000.0) -> (x/y=w425:dbl)
                    n130 = Multiply(x=w424, y=w425) -> (x*y=w423:dbl)
                    n131 = Divide(x=w423, y="Sinusoid period (s)") -> (x/y=w421:dbl)
                    n132 = Cosine(x=w421) -> (cos(x)=w420:dbl)
                    n133 = Multiply(x="Sinusoid amplitude (N)", y=w420) -> (x*y=w417:dbl)
                    n134 = Add(x=w418, y=w417) -> (x+y=w416:dbl)
                    n135 = local write "Single motor tension current set value"(w416) -> ()
                  }
                }
              }
            }
            n136 = case shown="True" "RecordTensionsForGivenTimeFlag" {
              selector: "RecordTensionsForGivenTimeFlag" -> [w314 w333]
              tunnel: [w314 w333] -> w294
              frame True {
                # "If we have recorded tensions for long \nenough, stop the recording by flipping \nthe record state flag to false."
                # "If the current recording state is different than the last state"
                # "In the ManualRecording = true state, \nkeep track of the recording time"
                n137 = local read "Manually record tensions flag previous state"() -> (w316:bool)
                n138 = Not Equal?(x=w314, y=w316) -> (x != y?=w315:bool)
                n139 = case shown="True" w315 {
                  tunnel: [w319 w325] -> w308
                  frame False {
                    n140 = Tick Count (ms)() -> (millisecond timer value=w319:u32)
                  }
                  frame True {
                    # "Create a manual recording file name\nwith hour_minute appended."
                    # "Mark start time of recording."
                    n141 = Tick Count (ms)() -> (millisecond timer value=w325:u32)
                    n142 = Format Date/Time String(time format string (%c)="%I", UTC format=FALSE) -> (date/time string=w329:string)  [unwired: 1 in]
                    n143 = Format Date/Time String(time format string (%c)="%M", UTC format=FALSE) -> (date/time string=w320:string)  [unwired: 1 in]
                    n144 = Divide(x=w325, y=1000.0) -> (x/y=→"StartManualTensionRecordTimeInSeconds":dbl)
                    n145 = Concatenate Strings("Manual_Tension_Record_" ("string"), w329, "_" ("string"), w320) -> (w324:string)
                    n146 = local write "Unity task info string"(w324) -> ()
                    n147 = local write "New info string received"(TRUE ("New info string received")) -> ()
                  }
                }
                n148 = local read "MaxTensionsRecordTimeInSecs"() -> (w310:dbl)
                n149 = local read "StartManualTensionRecordTimeInSeconds"() -> (w313:dbl)
                n150 = Divide(x=w308, y=1000.0) -> (x/y=w311:dbl)
                n151 = Subtract(x=w311, y=w313) -> (x-y=w307:dbl)
                "RecordTime (s)" <- w307
                n152 = Greater Or Equal?(x=w307, y=w310) -> (x >= y?=w309:bool)
                n153 = case shown="True" w309 {
                  frame False {
                  }
                  frame True {
                    n154 = local write "RecordTime (s)"(0.0 ("RecordTime (s)")) -> ()
                    n155 = local write "RecordTensionsForGivenTimeFlag"(FALSE ("RecordTensionsForGivenTimeFlag")) -> ()
                  }
                }
              }
              frame False {
                # "If the current recording state is different than the last state"
                n156 = local read "Manually record tensions flag previous state"() -> (w335:bool)
                n157 = Not Equal?(x=w333, y=w335) -> (x != y?=w334:bool)
                n158 = case shown="True" w334 {
                  frame False {
                  }
                  frame True {
                    # "If the recording flag just got set to false, then \nthe recording has ended."
                    n159 = local write "Task has ended flag"(TRUE ("Task has ended flag")) -> ()
                  }
                }
              }
            }
            "Manually record tensions flag previous state" <- w294
            n160 = case shown="True" "Live plot tensions flag" {
              tunnel: w297 -> [_ w373]
              tunnel: w292 -> [_ w337]
              frame False {
              }
              frame True {
                # "Send the tension data to the waveform plots for all tension sensors."
                n161 = Index Array(array=w337, index #1=0 ("index")) -> (element #1=w370:dbl, element #2=w381:dbl, element #3=w383:dbl, element #4=w385:dbl, element #5=w387:dbl, element #6=w389:dbl, element #7=w391:dbl, element #8=w396:dbl, element #9=w349:dbl, element #10=w347:dbl, element #11=w345:dbl, element #12=w343:dbl, element #13=w341:dbl, element #14=w339:dbl)  [unwired: 13 in]
                n162 = Index Array(array=w373, index #1=0 ("index")) -> (element #1=w371:dbl, element #2=w382:dbl, element #3=w384:dbl, element #4=w386:dbl, element #5=w388:dbl, element #6=w390:dbl, element #7=w392:dbl, element #8=w395:dbl, element #9=w348:dbl, element #10=w346:dbl, element #11=w344:dbl, element #12=w342:dbl, element #13=w340:dbl, element #14=w338:dbl)  [unwired: 13 in]
                n163 = Build Array(w370, w371) -> (w372:dbl[])
                n164 = Build Array(w381, w382) -> (w375:dbl[])
                n165 = Build Array(w383, w384) -> (w376:dbl[])
                n166 = Build Array(w385, w386) -> (w377:dbl[])
                n167 = Build Array(w387, w388) -> (w378:dbl[])
                n168 = Build Array(w389, w390) -> (w379:dbl[])
                n169 = Build Array(w391, w392) -> (w380:dbl[])
                n170 = Build Array(w396, w395) -> (w394:dbl[])
                n171 = Build Array(w349, w348) -> (w361:dbl[])
                n172 = Build Array(w347, w346) -> (w359:dbl[])
                n173 = Build Array(w345, w344) -> (w357:dbl[])
                n174 = Build Array(w343, w342) -> (w355:dbl[])
                n175 = Build Array(w341, w340) -> (w353:dbl[])
                n176 = Build Array(w339, w338) -> (w351:dbl[])
                n177 = Array To Cluster(array=w372) -> (cluster=→"1":cluster{"[0]":dbl, "[1]":dbl})
                n178 = Array To Cluster(array=w375) -> (cluster=→"2":cluster{"[0]":dbl, "[1]":dbl})
                n179 = Array To Cluster(array=w376) -> (cluster=→"3":cluster{"[0]":dbl, "[1]":dbl})
                n180 = Array To Cluster(array=w377) -> (cluster=→"4":cluster{"[0]":dbl, "[1]":dbl})
                n181 = Array To Cluster(array=w378) -> (cluster=→"5":cluster{"[0]":dbl, "[1]":dbl})
                n182 = Array To Cluster(array=w379) -> (cluster=→"6":cluster{"[0]":dbl, "[1]":dbl})
                n183 = Array To Cluster(array=w380) -> (cluster=→"7":cluster{"[0]":dbl, "[1]":dbl})
                n184 = Array To Cluster(array=w394) -> (cluster=→"8":cluster{"[0]":dbl, "[1]":dbl})
                n185 = Array To Cluster(array=w361) -> (cluster=→"9":cluster{"[0]":dbl, "[1]":dbl})
                n186 = Array To Cluster(array=w359) -> (cluster=→"10":cluster{"[0]":dbl, "[1]":dbl})
                n187 = Array To Cluster(array=w357) -> (cluster=→"11":cluster{"[0]":dbl, "[1]":dbl})
                n188 = Array To Cluster(array=w355) -> (cluster=→"12":cluster{"[0]":dbl, "[1]":dbl})
                n189 = Array To Cluster(array=w353) -> (cluster=→"13":cluster{"[0]":dbl, "[1]":dbl})
                n190 = Array To Cluster(array=w351) -> (cluster=→"14":cluster{"[0]":dbl, "[1]":dbl})
              }
            }
            n191 = case shown="True" "Capture current tension mean and standard dev" {
              frame False {
              }
              frame True {
                n192 = local read "All tensions standard dev"() -> (→"Captured tensions standard dev":dbl[])
                n193 = local read "All tensions mean"() -> (→"Captured tensions mean":dbl[])
              }
            }
          }
          event "Change constant tension value toggle": Value Change {
            n194 = event-data() -> ()  [unwired: 1 in, 6 out]
            n195 = local write "Single motor tension current set value"("Single motor tension desired set value") -> ()
          }
          event "Mode Pelvis": Value Change {
            n196 = event-data() -> ("NewVal"=w433:enum32{"Idle", "Constant", "Force", "Pert"})  [unwired: 1 in, 5 out]
            n197 = case shown="\"Pert\"" w433 {
              tunnel: [i16 0 ("Mode") i16 1 ("Mode") i16 2 ("Mode") i16 3 ("Mode")] -> w432
              frame "Idle", Default {
                n198 = property on="Mode Pelvis" class="RadioBtnsControl (strict)"() -> ("Controls[]"=w434:refnum<vi>[])  [unwired: 2 in, 2 out]
                n199 = Index Array(array=w434, index #1=1 ("index")) -> (element #1=w442:refnum<vi>, element #2=w436:refnum<vi>, element #3=w437:refnum<vi>)  [unwired: 2 in]
                n200 = property class="Ctl"(reference=w442, "DisabledEnum"=T7."Enabled" ("Disabled")) -> ()  [unwired: 1 in, 2 out]
                n201 = property class="Ctl"(reference=w436, "DisabledEnum"=T7."Disabled and Grayed Out" ("Disabled")) -> ()  [unwired: 1 in, 2 out]
                n202 = property class="Ctl"(reference=w437, "DisabledEnum"=T7."Disabled and Grayed Out" ("Disabled")) -> ()  [unwired: 1 in, 2 out]
              }
              frame "Constant" {
                n203 = property on="Mode Pelvis" class="RadioBtnsControl (strict)"() -> ("Controls[]"=w443:refnum<vi>[])  [unwired: 2 in, 2 out]
                n204 = Index Array(array=w443, index #1=0 ("index"), index #2=2 ("index"), index #3=3 ("index")) -> (element #1=w453:refnum<vi>, element #2=w445:refnum<vi>, element #3=w446:refnum<vi>)
                n205 = property class="Ctl"(reference=w453, "DisabledEnum"=T7."Enabled" ("Disabled")) -> ()  [unwired: 1 in, 2 out]
                n206 = property class="Ctl"(reference=w445, "DisabledEnum"=T7."Enabled" ("Disabled")) -> ()  [unwired: 1 in, 2 out]
                n207 = property class="Ctl"(reference=w446, "DisabledEnum"=T7."Enabled" ("Disabled")) -> ()  [unwired: 1 in, 2 out]
              }
              frame "Force" {
                n208 = property on="Mode Pelvis" class="RadioBtnsControl (strict)"() -> ("Controls[]"=w454:refnum<vi>[])  [unwired: 2 in, 2 out]
                n209 = Index Array(array=w454, index #1=0 ("index"), index #2=1 ("index"), index #3=3 ("index")) -> (element #1=w464:refnum<vi>, element #2=w456:refnum<vi>, element #3=w457:refnum<vi>)
                n210 = property class="Ctl"(reference=w464, "DisabledEnum"=T7."Disabled and Grayed Out" ("Disabled")) -> ()  [unwired: 1 in, 2 out]
                n211 = property class="Ctl"(reference=w456, "DisabledEnum"=T7."Enabled" ("Disabled")) -> ()  [unwired: 1 in, 2 out]
                n212 = property class="Ctl"(reference=w457, "DisabledEnum"=T7."Disabled and Grayed Out" ("Disabled")) -> ()  [unwired: 1 in, 2 out]
              }
              frame "Pert" {
                n213 = property on="Mode Pelvis" class="RadioBtnsControl (strict)"() -> ("Controls[]"=w465:refnum<vi>[])  [unwired: 2 in, 2 out]
                n214 = Index Array(array=w465, index #1=0 ("index"), index #2=1 ("index"), index #3=2 ("index")) -> (element #1=w475:refnum<vi>, element #2=w467:refnum<vi>, element #3=w468:refnum<vi>)
                n215 = property class="Ctl"(reference=w475, "DisabledEnum"=T7."Disabled and Grayed Out" ("Disabled")) -> ()  [unwired: 1 in, 2 out]
                n216 = property class="Ctl"(reference=w467, "DisabledEnum"=T7."Enabled" ("Disabled")) -> ()  [unwired: 1 in, 2 out]
                n217 = property class="Ctl"(reference=w468, "DisabledEnum"=T7."Disabled and Grayed Out" ("Disabled")) -> ()  [unwired: 1 in, 2 out]
              }
            }
            n218 = shared-variable "NI-PXIe8880-2F170198\\variables_AlwaysInUse - networkPublished.lvlib\\Mode_pelvis"(w432) -> ()  [unwired: 1 in, 1 out]
          }
          event Value Change {
            n219 = event-data() -> ("NewVal"=w477:T3)  [unwired: 1 in, 5 out]
            n220 = case shown="\"Pert\"" w477 {
              tunnel: [i16 0 ("Mode") i16 1 ("Mode") i16 2 ("Mode") i16 3 ("Mode")] -> w476
              frame "Idle", Default {
                n221 = property on="Mode Knees" class="RadioBtnsControl (strict)"() -> ("Controls[]"=w478:refnum<vi>[])  [unwired: 2 in, 2 out]
                n222 = Index Array(array=w478, index #1=1 ("index")) -> (element #1=w486:refnum<vi>, element #2=w480:refnum<vi>, element #3=w481:refnum<vi>)  [unwired: 2 in]
                n223 = property class="Ctl"(reference=w486, "DisabledEnum"=T7."Enabled" ("Disabled")) -> ()  [unwired: 1 in, 2 out]
                n224 = property class="Ctl"(reference=w480, "DisabledEnum"=T7."Disabled and Grayed Out" ("Disabled")) -> ()  [unwired: 1 in, 2 out]
                n225 = property class="Ctl"(reference=w481, "DisabledEnum"=T7."Disabled and Grayed Out" ("Disabled")) -> ()  [unwired: 1 in, 2 out]
              }
              frame "Constant" {
                n226 = property on="Mode Knees" class="RadioBtnsControl (strict)"() -> ("Controls[]"=w487:refnum<vi>[])  [unwired: 2 in, 2 out]
                n227 = Index Array(array=w487, index #1=0 ("index"), index #2=2 ("index"), index #3=3 ("index")) -> (element #1=w497:refnum<vi>, element #2=w489:refnum<vi>, element #3=w490:refnum<vi>)
                n228 = property class="Ctl"(reference=w497, "DisabledEnum"=T7."Enabled" ("Disabled")) -> ()  [unwired: 1 in, 2 out]
                n229 = property class="Ctl"(reference=w489, "DisabledEnum"=T7."Enabled" ("Disabled")) -> ()  [unwired: 1 in, 2 out]
                n230 = property class="Ctl"(reference=w490, "DisabledEnum"=T7."Enabled" ("Disabled")) -> ()  [unwired: 1 in, 2 out]
              }
              frame "Force" {
                n231 = property on="Mode Knees" class="RadioBtnsControl (strict)"() -> ("Controls[]"=w498:refnum<vi>[])  [unwired: 2 in, 2 out]
                n232 = Index Array(array=w498, index #1=0 ("index"), index #2=1 ("index"), index #3=3 ("index")) -> (element #1=w508:refnum<vi>, element #2=w500:refnum<vi>, element #3=w501:refnum<vi>)
                n233 = property class="Ctl"(reference=w508, "DisabledEnum"=T7."Disabled and Grayed Out" ("Disabled")) -> ()  [unwired: 1 in, 2 out]
                n234 = property class="Ctl"(reference=w500, "DisabledEnum"=T7."Enabled" ("Disabled")) -> ()  [unwired: 1 in, 2 out]
                n235 = property class="Ctl"(reference=w501, "DisabledEnum"=T7."Disabled and Grayed Out" ("Disabled")) -> ()  [unwired: 1 in, 2 out]
              }
              frame "Pert" {
                n236 = property on="Mode Knees" class="RadioBtnsControl (strict)"() -> ("Controls[]"=w509:refnum<vi>[])  [unwired: 2 in, 2 out]
                n237 = Index Array(array=w509, index #1=0 ("index"), index #2=1 ("index"), index #3=2 ("index")) -> (element #1=w519:refnum<vi>, element #2=w511:refnum<vi>, element #3=w512:refnum<vi>)
                n238 = property class="Ctl"(reference=w519, "DisabledEnum"=T7."Disabled and Grayed Out" ("Disabled")) -> ()  [unwired: 1 in, 2 out]
                n239 = property class="Ctl"(reference=w511, "DisabledEnum"=T7."Enabled" ("Disabled")) -> ()  [unwired: 1 in, 2 out]
                n240 = property class="Ctl"(reference=w512, "DisabledEnum"=T7."Disabled and Grayed Out" ("Disabled")) -> ()  [unwired: 1 in, 2 out]
              }
            }
            n241 = shared-variable "NI-PXIe8880-2F170198\\variables_AlwaysInUse - networkPublished.lvlib\\Mode_knees"(w476) -> ()  [unwired: 1 in, 1 out]
          }
          event "UseVicon": Value Change {
            n242 = event-data() -> ("NewVal"=w520:bool)  [unwired: 1 in, 5 out]
            n243 = Select(t=enum32{"Vicon", "no Vicon"}."Vicon", s=w520, f=enum32{"Vicon", "no Vicon"}."no Vicon") -> (s? t:f=→"ViconTab":enum32{"Vicon", "no Vicon"})
          }
          event "Connect\nVicon": Value Change {
            n244 = event-data() -> ()  [unwired: 1 in, 6 out]
            n245 = call "ConnectVicon.vi"("Mode"="Stream Mode") -> ("error out"=w533:errorcluster, "Connected"=→"Vicon Connected":bool, ".NET Refnum out"=w524:refnum<k24>)  [unwired: 8 in]
            n246 = disable-structure shown="Disabled" {
              frame Disabled {
                w543 = "."
                n247 = invoke class="Client" method="GetVersion"() -> ("GetVersion"=w548:refnum<k24>)  [unwired: 3 in, 2 out]
                n248 = property class="Output_GetVersion"(reference=w548) -> (reference out=w539:refnum<k24>, "Major"=w547:u32, "Minor"=w545:u32, "Point"=w546:u32)  [unwired: 1 in, 1 out]
                n249 = Close Reference(reference=w539) -> ()  [unwired: 1 in, 1 out]
                n250 = Number To Decimal String(number=w547) -> (decimal integer string=w544:string)  [unwired: 1 in]
                n251 = Number To Decimal String(number=w545) -> (decimal integer string=w541:string)  [unwired: 1 in]
                n252 = Number To Decimal String(number=w546) -> (decimal integer string=w542:string)  [unwired: 1 in]
                n253 = Concatenate Strings(w544, w543, w541, w543, w542) -> (→"SDK Version":string)
              }
              frame Enabled {
              }
            }
            n254 = invoke class="Client" method="GetFrame"(reference=w524, error in=w533) -> (reference out=w530:refnum<k24>, error out=w529:errorcluster)  [unwired: 1 in, 1 out]
            n255 = call "FrameNo.vi"("error in (no error)"=w529, ".NET Refnum in"=w530) -> ("error out"=w527:errorcluster, "FrameNumber"=w526:dbl, ".NET Reference out"=w528:refnum<k24>)  [unwired: 7 in]
            n256 = To Double Precision Float(number=w526) -> (double precision float=→"Frame Number":dbl)
            n257 = call "SubName.vi"("error in (no error)"=w527, ".NET Refnum in"=w528) -> ("error out"=w536:errorcluster, "SubjectName"=w534:string, ".NET Refnum out"=w531:refnum<k24>)  [unwired: 7 in]
            "Subject Name" <- w534
            n258 = call "Markers.vi"("error in (no error)"=w536, "Subject Name"=w534, ".NET Refnum in"=w531) -> ("Markers Count"=→"Markers Count":u32, ".NET Reference out"=→".NET Reference out":refnum<k24>)  [unwired: 5 in, 2 out]
          }
          event "Update\nMarkers": Value Change {
            n259 = event-data() -> ()  [unwired: 1 in, 6 out]
          }
          event "Vicon Static": Value Change {
            n260 = event-data() -> ()  [unwired: 1 in, 6 out]
          }
          event "Update Pert Parameters": Value Change {
            # "These are the Pert Parameters"
            n261 = event-data() -> ()  [unwired: 1 in, 6 out]
            n262 = shared-variable "NI-PXIe8880-2F170198\\Perturbation.lvlib\\Pert Direction"("Pert Direction") -> ()  [unwired: 1 in, 1 out]
            n263 = Multiply(x="Weight [Kg]", y=2.20462262) -> (x*y=→"Weight [lbs]":dbl)
            n264 = Divide(x="Amp [%BW]", y=100.0) -> (x/y=w555:dbl)
            n265 = Multiply(x="Weight [Kg]", y=9.98) -> (x*y=w554:dbl)
            n266 = Multiply(x=w555, y=w554) -> (x*y=w550:dbl)
            n267 = Build Array("Rise Time", "Constant Time", "Fall Time", w550) -> (w549:dbl[])
            n268 = shared-variable "NI-PXIe8880-2F170198\\Perturbation.lvlib\\Pert Param"(w549) -> ()  [unwired: 1 in, 1 out]
          }
          event "Update Pert Parameters 2": Value Change {
            n269 = event-data() -> ()  [unwired: 1 in, 6 out]
            n270 = shared-variable "NI-PXIe8880-2F170198\\Perturbation.lvlib\\Pert Direction_pel"("Pert Direction 2") -> ()  [unwired: 1 in, 1 out]
            n271 = Multiply(x="Weight [Kg] 3", y=2.20462262) -> (x*y=→"Weight [lbs] 3":dbl)
            n272 = Divide(x="Amp [%BW] 3", y=100.0) -> (x/y=w573:dbl)
            n273 = Multiply(x="Weight [Kg] 3", y=9.98) -> (x*y=w572:dbl)
            n274 = Multiply(x=w573, y=w572) -> (x*y=w571:dbl)
            n275 = Build Array("Rise Time 2", "Constant Time 2", "Fall Time 2", w571) -> (w564:dbl[])
            n276 = shared-variable "NI-PXIe8880-2F170198\\Perturbation.lvlib\\Pert Param 2"(w564) -> ()  [unwired: 1 in, 1 out]
          }
          event "Apply Pert": Value Change {
            n277 = event-data() -> ()  [unwired: 1 in, 6 out]
            n278 = shared-variable "NI-PXIe8880-2F170198\\ForceField.lvlib\\Apply Pert"("Apply Pert") -> ()  [unwired: 1 in, 1 out]
          }
          event "Apply Pert 2": Value Change {
            n279 = event-data() -> ()  [unwired: 1 in, 6 out]
            n280 = shared-variable "NI-PXIe8880-2F170198\\ForceField.lvlib\\Apply Pert_pel"("Apply Pert 2") -> ()  [unwired: 1 in, 1 out]
          }
          event "Refresh Center": Value Change {
            # "need to test"
            n281 = event-data() -> ()  [unwired: 1 in, 6 out]
            n282 = local read "trunk markers"() -> (w580:dbl[])
            n283 = shared-variable "NI-PXIe8880-2F170198\\ForceField.lvlib\\Refresh Center"("Refresh Center") -> ()  [unwired: 1 in, 1 out]
            n284 = call "getCenterpt.vi"("markers3"=w580) -> ("centerxyz"=w579:dbl[])  [unwired: 3 in]
            n285 = shared-variable "NI-PXIe8880-2F170198\\ForceField.lvlib\\trunk_cn"(w579) -> ()  [unwired: 1 in, 1 out]
          }
          event "Refresh Center 2": Value Change {
            n286 = event-data() -> ()  [unwired: 1 in, 6 out]
            n287 = flat-sequence {
              tunnel: [w585] -> w583
              tunnel: ["Refresh Center 2"] -> w582
              tunnel: w583 -> [w588]
              tunnel: w582 -> [w587]
              frame #0 {
                n288 = local read "pel markers"() -> (w586:dbl[])
                n289 = call "getCenterpt_pel.vi"("markers4"=w586) -> ("centerxyz"=w585:dbl[])  [unwired: 3 in]
              }
              frame #1 {
                n290 = shared-variable "NI-PXIe8880-2F170198\\ForceField.lvlib\\pel_cn"(w588) -> ()  [unwired: 1 in, 1 out]
                n291 = shared-variable "NI-PXIe8880-2F170198\\ForceField.lvlib\\Refresh Center_pel"(w587) -> ()  [unwired: 1 in, 1 out]
              }
            }
          }
          event "Pert Reset": Value Change {
            n292 = event-data() -> ()  [unwired: 1 in, 6 out]
            n293 = shared-variable "NI-PXIe8880-2F170198\\ForceField.lvlib\\Pert Reset"("Pert Reset") -> ()  [unwired: 1 in, 1 out]
          }
          event "Pert Reset 2": Value Change {
            n294 = event-data() -> ()  [unwired: 1 in, 6 out]
            n295 = shared-variable "NI-PXIe8880-2F170198\\ForceField.lvlib\\Pert Reset_pel"("Pert Reset 2") -> ()  [unwired: 1 in, 1 out]
          }
          event "Update R or FF": Value Change {
            n296 = event-data() -> ()  [unwired: 1 in, 6 out]
            n297 = shared-variable "NI-PXIe8880-2F170198\\ForceField.lvlib\\Radius"("Force Field Radius (m)") -> ()  [unwired: 1 in, 1 out]
            n298 = shared-variable "NI-PXIe8880-2F170198\\ForceField.lvlib\\Radius_Update"("Update R or FF") -> ()  [unwired: 1 in, 1 out]
            n299 = shared-variable "NI-PXIe8880-2F170198\\ForceField.lvlib\\FM --- FF"("FM --- FF") -> ()  [unwired: 1 in, 1 out]
            n300 = call "File Dialog"("start path"="Select File with Trunk\nBoundary Points") -> ("selected path"=w597:path)  [unwired: 11 in, 3 out]
            n301 = call-poly <vilib>:"Read Delimited Spreadsheet.vi"("file path (dialog if empty)"=w597, "delimiter (\\t)"="," ("delimiter (\\t)")) -> ("all rows"=w595:dbl[][])  [unwired: 8 in, 5 out]
            n302 = Index Array(array=w595, index (col)=0 ("disabled index (col)")) -> (element=w593:dbl[])  [unwired: 1 in]
            n303 = Index Array(array=w595, index (col)=1 ("disabled index (col)")) -> (element=w591:dbl[])  [unwired: 1 in]
            n304 = shared-variable "NI-PXIe8880-2F170198\\ForceField.lvlib\\Boundary X pts"(w593) -> ()  [unwired: 1 in, 1 out]
            n305 = shared-variable "NI-PXIe8880-2F170198\\ForceField.lvlib\\Boundary Y pts"(w591) -> ()  [unwired: 1 in, 1 out]
          }
          event "Update R or FF 2": Value Change {
            n306 = event-data() -> ()  [unwired: 1 in, 6 out]
            n307 = shared-variable "NI-PXIe8880-2F170198\\ForceField.lvlib\\FM --- FF_pel"("FM --- FF 2") -> ()  [unwired: 1 in, 1 out]
            n308 = shared-variable "NI-PXIe8880-2F170198\\ForceField.lvlib\\Radius_pel"("Pelvis Radius FF") -> ()  [unwired: 1 in, 1 out]
            n309 = shared-variable "NI-PXIe8880-2F170198\\ForceField.lvlib\\Radius_Update_pel"("Update R or FF 2") -> ()  [unwired: 1 in, 1 out]
            n310 = Divide(x="% Body Weight 2", y=100.0) -> (x/y=w610:dbl)
            n311 = Multiply(x="Weight (Kg) --- FF 2", y=9.81) -> (x*y=w607:dbl)
            n312 = Multiply(x=w607, y=w610) -> (x*y=w602:dbl)
            n313 = shared-variable "NI-PXIe8880-2F170198\\ForceField.lvlib\\K constant_pel"(w602) -> ()  [unwired: 1 in, 1 out]
          }
          event "record trajectory": Value Change {
            n314 = event-data() -> ()  [unwired: 1 in, 6 out]
          }
          event "Reset Label": Value Change {
            n315 = event-data() -> ()  [unwired: 1 in, 6 out]
            n316 = shared-variable "NI-PXIe8880-2F170198\\ForceField.lvlib\\downorUp"(FALSE) -> ()  [unwired: 1 in, 1 out]
          }
          event "Update_setForces": Value Change {
            n317 = event-data() -> ()  [unwired: 1 in, 6 out]
            n318 = shared-variable "NI-PXIe8880-2F170198\\ForceField.lvlib\\3D FF Parameters"("Set Unit Force Vector") -> ()  [unwired: 1 in, 1 out]
            n319 = Divide "kg"(x="Weight (lb)", y=2.205) -> (x/y=w621:dbl)
            n320 = Divide(x="Set % Body Weight", y=100.0) -> (x/y=w617:dbl)
            n321 = Multiply(x=w621, y=9.81) -> (x*y=w616:dbl)
            n322 = Multiply(x=w617, y=w616) -> (x*y=w615:dbl)
            n323 = shared-variable "NI-PXIe8880-2F170198\\ForceField.lvlib\\K constant_pel"(w615) -> ()  [unwired: 1 in, 1 out]
            n324 = shared-variable "NI-PXIe8880-2F170198\\ForceField.lvlib\\resetPelvicF"("Update_setForces") -> ()  [unwired: 1 in, 1 out]
          }
          event "Use ATI": Value Change {
            # "send to target"
            n325 = event-data() -> ("NewVal"=w624:bool)  [unwired: 1 in, 5 out]
            n326 = shared-variable "NI-PXIe8880-2F170198\\variables_AlwaysInUse - networkPublished.lvlib\\Use ATI"(w624) -> ()  [unwired: 1 in, 1 out]
            n327 = disable-structure shown="Disabled" {
              frame Disabled {
                # "Needs to be run one time as long the sensor is the same.\nIf sensor is changed, run this module ... generate the \nCalbMatrix and create a constant .... copy and paste in \nthe target program."
                n328 = call "ATICalbMatrix.vi"("Automation Refnum in"="ATIDAQFT._FTSensor") -> ()  [unwired: 9 in, 2 out]
              }
              frame Enabled {
              }
            }
          }
          event "ATI Bias": Value Change {
            n329 = event-data() -> ()  [unwired: 1 in, 6 out]
            n330 = shared-variable "NI-PXIe8880-2F170198\\variables_ATI - networkPublished.lvlib\\Bias"("ATI Bias") -> ()  [unwired: 1 in, 1 out]
          }
          event "ATI UnBias": Value Change {
            n331 = event-data() -> ()  [unwired: 1 in, 6 out]
            n332 = shared-variable "NI-PXIe8880-2F170198\\variables_ATI - networkPublished.lvlib\\UnBias"("ATI UnBias") -> ()  [unwired: 1 in, 1 out]
          }
          event "DataSave": Value Change {
            n333 = event-data() -> ("NewVal"=w628:bool)  [unwired: 1 in, 5 out]
            n334 = flat-sequence {
              tunnel: [w634] -> w629
              tunnel: w628 -> [w634]
              tunnel: w629 -> [w636]
              frame #0 {
                n335 = local read "Subject Name"() -> (w633:string)
                n336 = Concatenate Strings(w633, "_" ("string"), "Insert Test Name", ".txt" ("string")) -> (w635:string)
                "Current Filename" <- w635
                n337 = shared-variable "NI-PXIe8880-2F170198\\variables_SaveData - networkPublished.lvlib\\FileName"(w635) -> ()  [unwired: 1 in, 1 out]
              }
              frame #1 {
                n338 = shared-variable "NI-PXIe8880-2F170198\\variables_SaveData - networkPublished.lvlib\\SaveData"(w636) -> ()  [unwired: 1 in, 1 out]
              }
            }
          }
        }
      }
      n339 = node-c288(i64 10 ("Period"), 60000 ("Priority")) -> (w35:T8)  [unwired: 2 in]
      n340 = timed-loop {
        timing: w35 -> [_]
        timing-out: [_] -> w34
        stop <- w145 stop-if-true
        # "If (use cond.) TCP is valid, \nADD code to \ncheck to see if TCP\nis still valid. If not, change\nthe value. This will make code \ntry to reconnect when it drops"
        n341 = node-c288() -> (→"Finished Late? [i-1]":bool)  [unwired: 1 in, 3 out]
        n342 = local read "TCP connection to Unity?"() -> (w144:bool)
        n343 = case shown="False" w144 {
          frame False {
            n344 = local read "Control point data source"() -> (w149:T2)
            n345 = case shown="\"Unity\"" w149 {
              frame "None/Off", Default {
              }
              frame "Vicon" {
              }
              frame "Unity" {
                # "If not connected, keep updating the \nbase value for when the last message was \nreceived, so it is accurate when a \nconnection is made."
                n346 = TCP Open Connection(address="localhost", remote port or service name=u16 8052, error in (no error)=errorcluster {"status"=FALSE, "code"=0, "source"=""}) -> (connection ID=→"Unity TCP connection ID":refnum<k5>, error out=w151:errorcluster)  [unwired: 2 in]
                n347 = case shown="Error" w151 {
                  frame No Error {
                    n348 = local write "TCP connection to Unity?"(TRUE ("TCP connection to Unity?")) -> ()
                  }
                  frame Error {
                    # "TCP connection to Unity failed\n (perhaps a timeout or bad IP)"
                  }
                }
                n349 = Tick Count (ms)() -> (millisecond timer value=w150:u32)
                n350 = local write "LastTimeUnityTensionsReceivedInMs"(w150) -> ()
              }
            }
          }
          frame True {
            n351 = flat-sequence {
              frame #0 {
                n352 = case shown="\"Unity\"" "Control point data source" {
                  frame "None/Off", Default {
                  }
                  frame "Vicon" {
                  }
                  frame "Unity" {
                    # "Read a single ASCII message terminated with the \nCRLF character. Note: this will NOT flush the \nbuffer, as it only reads a single ASCII message."
                    # "Tokenize received \nstring"
                    n353 = local read "Unity TCP connection ID"() -> (w169:refnum<k5>)
                    n354 = TCP Read(connection ID=w169, bytes to read=1000, 7:T11."CRLF" ("mode (standard)"), 9:75 ("timeout ms (25000)")) -> (data out=w168:string)  [unwired: 1 in, 2 out]
                    n355 = call "Tokenize string on commas.vi"("Unity TCP data received"=w168) -> ("Tokenized Unity Message"=w170:string[])  [unwired: 10 in]
                    n356 = call "Parse_TCP_Message_From_Unity.vi"("Tokenized message string array"=w170) -> ("task Over Message Received Flag"=w158:bool, "Desired tensions by motor"=w161:T12, "Control point position coords"=w167:dbl[], "Command string"=w166:string, "Force field type specifier"=w163:string, "Center point of FF"=w165:dbl[], "File information string"=w159:string, "Trunk Structure Matrix"=w162:dbl[][], "Boundary points"=w164:dbl[])  [unwired: 6 in]
                    n357 = case shown="\"K\"" w166 {
                      tunnel: w167 -> [_ w174 _ _ _ _ _ _ _]
                      tunnel: w165 -> [_ _ w176 _ _ _ _ _ _]
                      tunnel: w164 -> [_ _ _ _ w180 _ _ _ _]
                      tunnel: w163 -> [_ _ _ w178 _ _ _ _ _]
                      tunnel: w162 -> [_ _ _ _ _ w183 _ _ _]
                      tunnel: w161 -> [_ _ _ _ _ _ w186 _ _]
                      tunnel: w159 -> [_ _ _ _ _ _ _ w214 _]
                      tunnel: w158 -> [_ _ _ _ _ _ _ _ w215]
                      frame "", Default {
                      }
                      frame "C" {
                        n358 = shared-variable "NI-PXIe8880-2F170198\\variables_Unity_Data.lvlib\\FF Control Point"(w174) -> (error out=w173:errorcluster)  [unwired: 1 in]
                        n359 = call <vilib>:"Flush Shared Variable Data.vi"("error in (no error)"=w173) -> ()  [unwired: 10 in, 1 out]
                        "Control point position coords" <- w174
                      }
                      frame "O" {
                        n360 = shared-variable "NI-PXIe8880-2F170198\\variables_Unity_Data.lvlib\\Center Point for FF"(w176) -> (error out=w175:errorcluster)  [unwired: 1 in]
                        n361 = call <vilib>:"Flush Shared Variable Data.vi"("error in (no error)"=w175) -> ()  [unwired: 10 in, 1 out]
                        "Center point for FF" <- w176
                      }
                      frame "F" {
                        # "Assign the force field type specifier string to the \nfront-panel display (for viewing) and to the \nnetwork-published var (for sending to PXI)"
                        n362 = shared-variable "NI-PXIe8880-2F170198\\variables_Unity_Data.lvlib\\Force Field Type Specifier"(w178) -> (error out=w177:errorcluster)  [unwired: 1 in]
                        n363 = call <vilib>:"Flush Shared Variable Data.vi"("error in (no error)"=w177) -> ()  [unwired: 10 in, 1 out]
                        "Trunk FF type specifier" <- w178
                      }
                      frame "E" {
                        n364 = shared-variable "NI-PXIe8880-2F170198\\variables_Unity_Data.lvlib\\Excursion Distances Vicon Frame"(w180) -> (error out=w179:errorcluster)  [unwired: 1 in]
                        n365 = call <vilib>:"Flush Shared Variable Data.vi"("error in (no error)"=w179) -> ()  [unwired: 10 in, 1 out]
                        "Excursion distances Vicon frame" <- w180
                      }
                      frame "T" {
                        # "We pass the S matrix as a 1D array, since we\ncannot use 2D arrays as network-published \nvariables. NOTE: since we must specify the \nnumber of elements, this is our current limitation\non flexibly choosing the number of motors per belt."
                        n366 = Reshape Array(w183, 24 ("dimension size")) -> (w182:dbl[])
                        n367 = shared-variable "NI-PXIe8880-2F170198\\variables_Unity_Data.lvlib\\Trunk Structure Matrix"(w182) -> (error out=w181:errorcluster)  [unwired: 1 in]
                        n368 = call <vilib>:"Flush Shared Variable Data.vi"("error in (no error)"=w181) -> ()  [unwired: 10 in, 1 out]
                        "Trunk Structure Matrix" <- w183
                      }
                      frame "K" {
                        n369 = flat-sequence {
                          tunnel: w186 -> [w199]
                          tunnel: [w189] -> w185
                          tunnel: w185 -> [w212]
                          frame #0 {
                            # "\"K\" is the primary update tensions command. \nMost other messages are no longer used. \nOther still-used message headers: \n\"I\" = information (about subject, date, time)"
                            # "In for loop, we subtract 1 \nfrom motor index because\nLabview is zero-indexed."
                            # "Motors for which a desired tension value were sent \nare put into the array at their corresponding index. \nMotors without specified tension values are set to 0.\nResult = an ordered array (motors 1-14) with desired tensions."
                            n370 = Unbundle By Name(w199) -> ("Most Recent Vicon Frame Number"=w188:u32, "Corresponding motor tensions"=w196:dbl[], "Motor numbers"=w198:i32[])
                            "Last Vicon Frame Read" <- w188
                            n371 = Initialize Array(0.0 ("element"), "Total Number Motors") -> (w197:dbl[])
                            n372 = for {
                              tunnel: w198 -> [w204] mode=indexing
                              shift-right: [w205] -> w195
                              shift-left: w197 -> [w207]
                              tunnel: w196 -> [w206] mode=indexing
                              n373 = Subtract(x=w204, y=1) -> (x-y=w202:i32)
                              n374 = Replace Array Subset(array=w207, new element=w206, index=w202) -> (w205:dbl[])
                            }
                            "UnityDesiredCableTensionsInAscendingOrder" <- w195
                            n375 = shared-variable "NI-PXIe8880-2F170198\\variables_Unity_Data.lvlib\\MostRecentViconFrameNumber"(w188) -> ()  [unwired: 1 in, 1 out]
                            n376 = local read "LastTimeUnityTensionsReceivedInMs"() -> (w194:u32)
                            n377 = Tick Count (ms)() -> (millisecond timer value=w189:u32)
                            n378 = Subtract(x=w189, y=w194) -> (x-y=w193:u32)
                            n379 = Divide(x=w193, y=u32 1000) -> (x/y=w191:dbl)
                            n380 = Divide(x=1.0, y=w191) -> (x/y=→"TensionsUpdateRateHz":dbl)
                          }
                          frame #1 {
                            # "Flush the TCP buffer by reading a \nlarge amount of bytes in \nStandard Mode."
                            # "This frame is needed (ugh) to track\nthe update rate for receiving the \n\"K\" (update tensions) command."
                            n381 = local read "Unity TCP connection ID"() -> (w208:refnum<k5>)
                            n382 = TCP Read(connection ID=w208, bytes to read=500, 7:T11."Standard" ("mode (standard)"), 9:1 ("timeout ms (25000)")) -> ()  [unwired: 1 in, 3 out]
                            "LastTimeUnityTensionsReceivedInMs" <- w212
                          }
                        }
                      }
                      frame "I" {
                        "Unity task info string" <- w214
                        "New info string received" <- TRUE ("New info string received")
                      }
                      frame "S" {
                        "Task has ended flag" <- w215
                      }
                    }
                  }
                }
              }
            }
          }
        }
        n383 = node-c288() -> ()  [unwired: 1 in, 1 out]
        n384 = local read "Stop"() -> (w145:bool)
      }
      n385 = node-c288(w37) -> ()  [unwired: 1 out]
      n386 = node-c288(i64 10 ("Period"), 1 ("Priority")) -> (w28:T8)  [unwired: 7 in]
      n387 = timed-loop {
        timing: w28 -> [_]
        timing-out: [_] -> w27
        stop <- w39 stop-if-true
        n388 = node-c288() -> ()  [unwired: 1 in, 1 out]
        n389 = flat-sequence {
          tunnel: [w75] -> w39
          frame #0 {
            # "For each column, which is \nthe history for one sensor."
            # "Compute and store tension sensor \nstandard deviation."
            # "Below: store tension history\nin a local variable and compute \nstandard deviation of tension \nsensor history."
            # "We record only when we are connected to Unity."
            n390 = shared-variable "NI-PXIe8880-2F170198\\variables_Unity_Data.lvlib\\DesiredTensionsInAscendingMotorOrder"() -> (w60:dbl[])  [unwired: 1 in, 1 out]
            n391 = local read "All tensions history"() -> (w52:dbl[][])
            n392 = local read "Unity task info string"() -> (w67:string)
            n393 = local read "Task has ended flag"() -> (w61:bool)
            n394 = local read "New info string received"() -> (w65:bool)
            n395 = Array Size(array=w52) -> (size(s)=w54:i32[])
            n396 = local read "Connected to Unity last save call?"() -> (w63:bool)
            n397 = shared-variable "NI-PXIe8880-2F170198\\variables_Unity_Data.lvlib\\AllCurrentTensions"() -> (w49:dbl[])  [unwired: 1 in, 1 out]
            n398 = Index Array(array=w54, index=1) -> (element=w45:i32)
            n399 = Index Array(array=w54, index=0) -> (element=w47:i32)
            n400 = local read "Last Vicon Frame Read"() -> (w66:u32)
            n401 = local read "TCP connection to Unity?"() -> (w74:bool)
            n402 = Subtract(x=w47, y=1.0) -> (x-y=w56:dbl)
            n403 = local read "Current save file out"() -> (w71:path)
            n404 = Array Subset(array=w52, index (row)=0 ("index"), length (row)=w56, index (col)=0 ("index"), length (col)=w45) -> (w51:dbl[][])
            n405 = local read "Data to save"() -> (w68:dbl[][])
            n406 = call "write_markerdata.vi"("Data to save in"=w68, "Connected to Unity last call? In"=w63, "Connected to Unity via TCP?"=w74, "Host folder"=path "C:/Users/ROAR/Documents/Rob Motor Assessment stuff/Labview/RobUST_3D_with_Unity_Control_PXI_Low_Level_Only_Streamlined/Recorded_Data", "Unity task info string"=w67, "DesiredTensions"=w60, "Current save file in"=w71, "CurrentTensions"=w49, "New task info string flag in"=w65, "Last Vicon frame read"=w66, "Task has ended flag"=w61) -> ("Connected to Unity last call? Out"=→"Connected to Unity last save call?":bool, "Current save file out"=→"Current save file out":path, "Data to save"=→"Data to save":dbl[][], "New task info string flag out"=w64:bool, "Task had ended flag out"=w62:bool)  [unwired: 4 in]
            n407 = local read "Stop"() -> (w75:bool)
            n408 = Insert Into Array(array=w51, index (row)=0, new element=w49) -> (w48:dbl[][])  [unwired: 1 in]
            n409 = local write "New info string received"(w64) -> ()
            n410 = local write "All tensions history"(w48) -> ()
            n411 = local read "All tensions standard dev"() -> (w46:dbl[])
            n412 = local read "All tensions mean"() -> (w43:dbl[])
            n413 = local write "Task has ended flag"(w62) -> ()
            n414 = for {
              N: w45 -> [_]
              shift-right: [w80] -> _
              shift-left: w48 -> [w80]
              tunnel: w45 -> [_]
              shift-right: [w81] -> w44
              shift-left: w46 -> [w83]
              shift-right: [w76] -> w42
              shift-left: w43 -> [w77]
              i -> [w79]
              n415 = Index Array(array=w80, index (col)=w79) -> (element=w84:dbl[])  [unwired: 1 in]
              n416 = call <vilib>:"Std Deviation and Variance.vi"("X"=w84) -> ("mean"=w78:dbl, "standard deviation"=w82:dbl)  [unwired: 1 in, 1 out]
              n417 = Replace Array Subset(array=w77, new element=w78, index=w79) -> (w76:dbl[])
              n418 = Replace Array Subset(array=w83, new element=w82, index=w79) -> (w81:dbl[])
            }
            "All tensions mean" <- w42
            n419 = local write "All tensions standard dev"(w44) -> ()
          }
          frame #1 {
            n420 = Wait (ms)(milliseconds to wait=u32 20) -> ()  [unwired: 1 out]
          }
        }
        n421 = node-c288() -> ()  [unwired: 1 in, 1 out]
      }
      n422 = node-c288(w27) -> ()  [unwired: 1 out]
      n423 = node-c288(i64 5 ("Period")) -> (w31:T8)  [unwired: 3 in]
      n424 = timed-loop {
        timing: w31 -> [_]
        timing-out: [_] -> w30
        stop <- _ stop-if-true
        # "The only way to reliably check if a TCP connection\nis still open is to see the last time we got data. If it \nhas been more than 50 ms since we received a \"K\"\ncommand, close the TCP connection."
        n425 = node-c288() -> ()  [unwired: 1 in, 1 out]
        n426 = local read "LastTimeUnityTensionsReceivedInMs"() -> (w133:u32)
        n427 = Tick Count (ms)() -> (millisecond timer value=w134:u32)
        n428 = Subtract(x=w134, y=w133) -> (x-y=w132:u32)
        n429 = Greater?(x=w132, y=u32 3000) -> (0:w130:bool)
        n430 = case shown="True" w130 {
          frame False {
          }
          frame True {
            n431 = local read "Unity TCP connection ID"() -> (w135:refnum<k5>)
            n432 = local write "TCP connection to Unity?"(FALSE ("TCP connection to Unity?")) -> ()
            n433 = TCP Close Connection(connection ID=w135) -> ()  [unwired: 2 in, 2 out]
          }
        }
        n434 = node-c288() -> ()  [unwired: 1 in, 1 out]
      }
      n435 = node-c288(w34) -> ()  [unwired: 1 out]
      n436 = node-c288(w30) -> ()  [unwired: 1 out]
    }
  }
